vi "VI Tree.vi"   [LabVIEW 2018]
uses:
  app/solar_app_ctl Info.ctl
  excel/solar_excel_ctl TSV.ctl
  excel/solar_excel_ctl App.ctl
  excel/solar_excel_ctl Format.ctl
  excel/solar_excel_ctl Workbook.ctl
  excel/solar_excel_ctl Worksheet.ctl
  misc/solar_misc_ctl Email Config.ctl
  qtimer/solar_qtimer_ctl QTimer Settings.ctl
  qtimer/solar_qtimer_ctl QTimer.ctl
  qtimer/solar_qtimer_ctl Refnum.ctl
  qtimer/solar_qtimer_ctl SEQ.ctl
  solar/solar.lvclass
  voyager/solar_voy_ctl Voyager Refnum.ctl
  solar/solar_ctl Target Global.ctl
  solar/solar_ctl SOLAR Global.ctl
  solar/solar_ctl SOLAR Refnum.ctl
  solar/solar_ctl SOLAR UI Panes.ctl
  tcp/solar_tcp_ctl Action.ctl
  tcp/solar_tcp_ctl Config.ctl
  tcp/solar_tcp_ctl Debug.ctl
  tcp/solar_tcp_ctl Data.ctl
  type/solar_type Item Type.ctl
  type/solar_type Item.ctl
  voyager/solar_voy_def/solar_voy_def_ctl HANDSHAKE.ctl
  voyager/solar_voy_def/solar_voy_def_ctl ITEM TYPE.ctl
  voyager/solar_voy_def/solar_voy_def_ctl ITEM.ctl
  voyager/solar_voy_def/solar_voy_def_ctl HDR.ctl
  voyager/solar_voy_def/solar_voy_def_ctl INTERFACE (LINC).ctl
  voyager/solar_voy_def/solar_voy_def_ctl INTERFACE.ctl
  voyager/solar_voy_def/solar_voy_def_ctl ITEM (Simple).ctl
  voyager/solar_voy_def/solar_voy_def_ctl MODIFIERS CONVERSION.ctl
  voyager/solar_voy_def/solar_voy_def_ctl MODIFIERS LIMITS.ctl
  voyager/solar_voy_def/solar_voy_def_ctl MODIFIERS STATE.ctl
  voyager/solar_voy_def/solar_voy_def_ctl MODIFIERS UNITS.ctl
  voyager/solar_voy_def/solar_voy_def_ctl MODIFIERS.ctl
  voyager/solar_voy_def/solar_voy_def_ctl PACKET_ID.ctl
  voyager/solar_voy_def/solar_voy_def_ctl PACKET.ctl
  voyager/solar_voy_def/solar_voy_def_ctl PATH.ctl
  voyager/solar_voy_ctl Port Setup.ctl
  voyager/solar_voy_ctl Port.ctl
  voyager/solar_voy_ctl Setup.ctl
  voyager/solar_voy_ctl TCP.ctl
  voyager/solar_voy_ctl Voyager.ctl
types:
  T1 = cluster{"Native COSMOS Packets":cluster{"MYUINT8":cluster{"VALUE":u8}, "MYUINT16":cluster{"VALUE":u16}, "MYUINT32":cluster{"VALUE":u32}, "MYUINT64":cluster{"VALUE":u64}, "MYINT8":cluster{"VALUE":i8}, "MYINT16":cluster{"VALUE":i16}, "MYINT32":cluster{"VALUE":i32}, "MYINT64":cluster{"VALUE":i64}, "MYFLOAT32":cluster{"VALUE":sgl}, "MYFLOAT64":cluster{"VALUE":dbl}, "MYSTRING":cluster{"VALUE":string}, "MYBLOCK":cluster{"VALUE,t=block":string}}, "Native COSMOS Array Packets":cluster{"MYUINT8_1D":cluster{"VALUE":u8[]}, "MYUINT16_1D":cluster{"VALUE":u16[]}, "MYUINT32_1D":cluster{"VALUE":u32[]}, "MYUINT64_1D":cluster{"VALUE":u64[]}, "MYINT8_1D":cluster{"VALUE":i8[]}, "MYINT16_1D":cluster{"VALUE":i16[]}, "MYINT32_1D":cluster{"VALUE":i32[]}, "MYINT64_1D":cluster{"VALUE":i64[]}, "MYFLOAT32_1D":cluster{"VALUE":sgl[]}, "MYFLOAT64_1D":cluster{"VALUE":dbl[]}, "MYSTRING_1D":cluster{"VALUE":string[]}, "MYBLOCK_1D":cluster{"VALUE,t=block":string[]}}, "Native COSMOS Array Packets Fixed":cluster{"MYUINT8_1D":cluster{"VALUE,b=24":u8[]}, "MYUINT16_1D":cluster{"VALUE,b=48":u16[]}, "MYUINT32_1D":cluster{"VALUE,b=96":u32[]}, "MYUINT64_1D":cluster{"VALUE,b=192":u64[]}, "MYINT8_1D":cluster{"VALUE,b=24":i8[]}, "MYINT16_1D":cluster{"VALUE,b=48":i16[]}, "MYINT32_1D":cluster{"VALUE,b=96":i32[]}, "MYINT64_1D":cluster{"VALUE,b=192":i64[]}, "MYFLOAT32_1D":cluster{"VALUE,b=128":sgl[]}, "MYFLOAT64_1D":cluster{"VALUE,b=256":dbl[]}, "MYSTRING_1D":cluster{"VALUE,b=352,e=88":string[]}, "MYBLOCK_1D":cluster{"VALUE,t=block,b=192,e=48":string[]}}, "Custom LabVIEW Packets":cluster{"MYUINT8_ENUM":cluster{"VALUE":enum8{"ITEM1", "ITEM2", "ITEM3"}}, "MYUINT16_ENUM":cluster{"VALUE":enum16{"CAT", "DOG", "BIRD", "MOOSE"}}, "MYUINT32_ENUM":cluster{"VALUE":enum32{"ryan", "susan", "steve", "larry", "smith", "joe"}}, "MYBOOLEAN":cluster{"VALUE,s=OFF|ON":bool}, "MYSTRING_FIXED":cluster{"VALUE,b=24":string}, "MYBLOCK_FIXED":cluster{"VALUE,t=block,b=32":string}, "MYPATH":cluster{"VALUE":path}}, "Custom Test Packets":cluster{"MYTEST1":cluster{"MYFLOAT64":dbl, "MYSTRING":string}, "MYTEST2":cluster{"MYFLOAT64":dbl, "MYBLOCK,t=block":string}, "MYTEST3":cluster{"MYBOOLEAN,s=OK|ERROR":bool, "MYI32":i32, "MYSTRING":string}, "TEST_PACKET":cluster{"U32_COUNTER":u32, "DBL_NUMBER":dbl, "STRING,b=480":string, "BOOLEAN":bool, "U16_ENUM":enum16{"ENUM_ONE", "ENUM_TWO", "ENUM_THREE"}, "U8_RING":u8, "U32_ARRAY,e=5":u32[], "U8":u32}}}
  T2 = typedef "solar_voy_ctl Voyager.ctl" = cluster{"PACKETS":T3[], "COSMOS_Root":path, "CMD_HDR":T8, "TLM_HDR":T8, "TCPs":T9[], "VoyagerIDOffset":cluster{"VoyagerIDOffset":u16[], "Target Names":string[]}}
  T3 = typedef "solar_voy_def_ctl PACKET.ctl" = cluster{"PACKET_ID":T4, "ENDIAN":enum8{"BIG", "LITTLE"}, "DESC":string, "HZRD":bool, "ITEMS":T5[], "NoExport":bool, "last_time":timestamp, "last_count":u32, "last_data":string}
  T4 = typedef "solar_voy_def_ctl PACKET_ID.ctl" = cluster{"ID":u16, "CMD":enum8{"CMD", "TLM"}, "TARGET":string, "PACKET":string}
  T5 = typedef "solar_voy_def_ctl ITEM.ctl" = cluster{"NAME":string, "OFFSET":i32, "SIZE":i32, "TYPE":T6, "EACH_SIZE":i32, "LVTYPE":T7, "MIN":dbl, "MAX":dbl, "DEFAULT":string, "DESC":string, "ID":bool, "MODIFIERS":variant, "last_value":variant}
  T6 = typedef "solar_voy_def_ctl ITEM TYPE.ctl" = enum8{"BLOCK", "INT", "UINT", "FLOAT", "STRING"}
  T7 = typedef "solar_type Item Type.ctl" = enum16{"NULL", "UNKNOWN", "CLUSTER", "I8", "I16", "I32", "I64", "U8", "U16", "U32", "U64", "U8_ENUM", "U16_ENUM", "U32_ENUM", "SGL", "DBL", "BOOLEAN", "STRING", "PATH", "VISA", "TAG", "TIME", "I8_1D", "I16_1D", "I32_1D", "I64_1D", "U8_1D", "U16_1D", "U32_1D", "U64_1D", "U8_ENUM_1D", "U16_ENUM_1D", "U32_ENUM_1D", "SGL_1D", "DBL_1D", "BOOLEAN_1D", "STRING_1D", "PATH_1D", "VISA_1D", "TAG_1D", "TIME_1D", "I8_2D", "I16_2D", "I32_2D", "I64_2D", "U8_2D", "U16_2D", "U32_2D", "U64_2D", "U8_ENUM_2D", "U16_ENUM_2D", "U32_ENUM_2D", "SGL_2D", "DBL_2D", "BOOLEAN_2D", "STRING_2D", "PATH_2D", "VISA_2D", "TAG_2D", "TIME_2D"}
  T8 = typedef "solar_voy_def_ctl HDR.ctl" = cluster{"ITEMS":T5[], "LENGTH_NAME":string, "LENGTH_VALUE_OFFSET":i32, "ID_NAME":string, "ENDIAN":enum8{"BIG", "LITTLE"}, "GUID_NAME":string, "DEFAULT_TARGET":string, "DEFAULT_PACKET":string, "DEFAULT_ERROR":string}
  T9 = typedef "solar_voy_ctl TCP.ctl" = cluster{"Connected":bool, "Port":u16, "Listener":refnum<k5>, "ServerIP":string, "TCP":refnum<k5>, "Setup":T10, "VIRefnum":refnum<vi>, "TARGETS_CMD":string[], "TARGETS_TLM":string[]}
  T10 = typedef "solar_voy_ctl Port Setup.ctl" = enum8{"SERVER", "CLIENT", "SERVER_CMD", "SERVER_TLM"}
  T11 = typedef "solar_voy_ctl Voyager Refnum.ctl" = refnum<k1>
  T12 = typedef "solar_voy_ctl Setup.ctl" = cluster{"HEADER":enum8{"LINC", "CCSDS"}, "COSMOS_ROOT":path, "DEFAULT_TARGET":string}
  T13 = typedef "solar_voy_ctl Port.ctl" = cluster{"Setup":T10, "Port":u16, "ServerIP":string, "Target":string}
  T14 = typedef "solar_voy_def_ctl PATH.ctl" = enum8{"..", "config", "config/data", "config/system", "config/targets", "config/targets/TARGET", "config/targets/TARGET/cmd_tlm", "config/targets/TARGET/lib", "config/targets/TARGET/screens", "config/tools", "config/tools/cmd_tlm_server", "config/tools/data_viewer", "config/tools/handbook_creator", "config/tools/launcher", "config/tools/limits_monitor", "config/tools/opengl_builder", "config/tools/script_runner", "config/tools/table_manager", "config/tools/test_runner", "config/tools/tlm_extractor", "config/tools/tlm_grapher", "config/tools/tlm_viewer", "lib", "outputs", "outputs/handbooks", "outputs/logs", "outputs/saved_config", "outputs/tables", "outputs/tmp", "procedures", "tools", "Launcher.bat", "config/system/system.txt", "config/targets/TARGET/cmd_tlm/TARGET_cmd.txt", "config/targets/TARGET/cmd_tlm/TARGET_tlm.txt", "config/targets/TARGET/cmd_tlm_server.txt", "config/targets/TARGET/target.txt", "config/tools/cmd_tlm_server/cmd_tlm_server.txt", "config/tools/data_viewer/data_viewer.txt", "config/tools/handbook_creator/handbook_creator.txt", "config/tools/launcher/launcher.txt", "config/tools/limits_monitor/limits_monitor.txt", "config/tools/opengl_builder/opengl_builder.txt", "config/tools/script_runner/script_runner.txt", "config/tools/table_manager/table_manager.txt", "config/tools/test_runner/test_runner.txt", "config/tools/tlm_extractor/tlm_extractor.txt", "config/tools/tlm_grapher/tlm_grapher.txt", "config/tools/tlm_viewer/tlm_viewer.txt"}
  T15 = typedef "solar_voy_def_ctl MODIFIERS.ctl" = cluster{"LIMITS":T16, "UNITS":T17, "STATES":T18[], "CONVERSION":T19, "FORMAT":string, "REQUIRED":bool, "META":string[][]}
  T16 = typedef "solar_voy_def_ctl MODIFIERS LIMITS.ctl" = cluster{"NAME":string, "PERSIST":i32, "EN":bool, "RED_LO":dbl, "YEL_LO":dbl, "YEL_HI":dbl, "RED_HI":dbl, "GRN_LO":dbl, "GRN_HI":dbl, "FILENAME":string, "ARGS":string}
  T17 = typedef "solar_voy_def_ctl MODIFIERS UNITS.ctl" = cluster{"FULL":string, "ABV":string}
  T18 = typedef "solar_voy_def_ctl MODIFIERS STATE.ctl" = cluster{"KEY":string, "VALUE":string, "COLOR":string, "DESC":string, "HZRD":bool}
  T19 = typedef "solar_voy_def_ctl MODIFIERS CONVERSION.ctl" = cluster{"GENERIC":string, "FILENAME":string, "ARGS":string, "POLYS":cluster{"SEG":bool, "POLY":dbl[]}[]}
  T20 = typedef "solar_voy_def_ctl ITEM (Simple).ctl" = cluster{"NAME":string, "LVTYPE":T7, "BIT_SIZE":i32, "TYPE":T6, "DEFAULT":string, "EACH_SIZE":i32, "ID":bool, "STATES(k,v)":string[][], "DESC":string}
  T21 = typedef "solar_voy_def_ctl INTERFACE.ctl" = cluster{"INTERFACE":string, "TARGETS":string[], "Other":string[]}
  T22 = typedef "solar_voy_def_ctl INTERFACE (LINC).ctl" = cluster{"name":string, "hostname":string, "port":u16, "handshake_enabled":bool, "response_timeout":dbl, "read_timeout":dbl, "write_timeout":dbl, "length_bitoffset":i32, "length_bitsize":i32, "length_value_offset":i32, "fieldname_guid":string, "endianness":enum8{"BIG", "LITTLE"}, "fieldname_cmd_length":string, "Targets":string[]}
  T23 = typedef "solar_voy_def_ctl HANDSHAKE.ctl" = cluster{"ORIGIN":enum8{"RMT", "LCL"}, "STATUS,s=OK,ERROR":bool, "CODE":i32, "TIME_SECONDS":u32, "TIME_MICROSECONDS":u32, "DATA,t=BLOCK":string}
  T24 = typedef "solar_type Item.ctl" = cluster{"Item":string, "Type":T7, "Value":variant, "States":string[]}
  T25 = cluster{"U8":u8, "U16":u16, "U32":u32, "U64":u64, "I8":i8, "I16":i16, "I32":i32, "I64":i64, "U8_ENUM":enum8{"ITEM1", "ITEM2", "ITEM3"}, "U16_ENUM":enum16{"ITEM1", "ITEM2", "ITEM3"}, "U32_ENUM":enum32{"ITEM1", "ITEM2", "ITEM3"}, "SGL":sgl, "DBL":dbl, "BOOLEAN":bool, "STRING":string, "PATH":path, "VISA":refnum<visa-resource-name>, "TAG":tag, "TIME":timestamp, "U8_1D":u8[], "U16_1D":u16[], "U32_1D":u32[], "U64_1D":u64[], "I8_1D":i8[], "I16_1D":i16[], "I32_1D":i32[], "I64_1D":i64[], "U8_ENUM_1D":enum8{"ITEM1", "ITEM2", "ITEM3"}[], "U16_ENUM_1D":enum16{"ITEM1", "ITEM2", "ITEM3"}[], "U32_ENUM_1D":enum32{"ITEM1", "ITEM2", "ITEM3"}[], "SGL_1D":sgl[], "DBL_1D":dbl[], "STRING_1D":string[], "PATH_1D":path[], "VISA_1D":refnum<visa-resource-name>[], "TAG_1D":tag[], "TIME_1D":timestamp[], "U8_2D":u8[][], "U16_2D":u16[][], "U32_2D":u32[][], "U64_2D":u64[][], "I8_2D":i8[][], "I16_2D":i16[][], "I32_2D":i32[][], "I64_2D":i64[][], "U8_ENUM_2D":enum8{"ITEM1", "ITEM2", "ITEM3"}[][], "U16_ENUM_2D":enum16{"ITEM1", "ITEM2", "ITEM3"}[][], "U32_ENUM_2D":enum32{"ITEM1", "ITEM2", "ITEM3"}[][], "SGL_2D":sgl[][], "DBL_2D":dbl[][], "STRING_2D":string[][], "PATH_2D":path[][], "VISA_2D":refnum<visa-resource-name>[][], "TAG_2D":tag[][], "TIME_2D":timestamp[][]}
  T26 = typedef "solar_tcp_ctl Debug.ctl" = cluster{"Time":timestamp, "Action":T27, "ID":string, "Message":string, "Error":string, "Clients":string}
  T27 = typedef "solar_tcp_ctl Action.ctl" = enum16{"Decide", "CreateListener", "Open", "Read", "Write", "Close", "Shutdown", "Done", "ChangePort"}
  T28 = typedef "solar_tcp_ctl Data.ctl" = cluster{"Connected":bool, "Config":T29, "Clients":cluster{"Address":string, "Port":u16, "Valid":bool, "ClientID":refnum<k5>}[], "ConnectionID":refnum<k5>, "Debug":T26[]}
  T29 = typedef "solar_tcp_ctl Config.ctl" = cluster{"TCPServer":enum8{"SERVER", "CLIENT"}, "ServerPort":u16, "IPAddress":string, "ClientPort":u16, "HdrSizeBytes":i32, "HdrLenSubtractBytes":i32, "HdrLenOffsetBits":i32, "HdrLenSizeBits":i32}
  T30 = typedef "solar_ctl Target Global.ctl" = cluster{"Target":string, "Q":refnum<queue>, "UE":refnum<user-event>, "VI":refnum<vi>, "Menu":refnum<k9>, "Data":refnum<data-value>, "Attributes":variant}
  T31 = typedef "solar_ctl SOLAR UI Panes.ctl" = cluster{"Status":bool, "Emergency":bool, "Targets":bool}
  T32 = typedef "solar_ctl SOLAR Refnum.ctl" = refnum<k1>
  T33 = typedef "solar_ctl SOLAR Global.ctl" = cluster{"Targets":T30[], "AppDir":path, "solar.ini":path, "ConfigsDir":path, "CosmosDir":path, "LogsDir":path, "ExePath":path, "ExeVersion":string, "PartNum":string, "AppSetup":string, "Title":string, "Main.ini":path, "Temp.ini":path, "vSOLAR":string, "Splash.png":string, "SplashWait":i32, "SOLARUE":refnum<user-event>, "VoyagerRefnum":T11, "QTimerRefnum":T34}
  T34 = typedef "solar_qtimer_ctl Refnum.ctl" = refnum<k1>
  T35 = typedef "solar_qtimer_ctl SEQ.ctl" = cluster{"QTimers":T36[]}
  T36 = typedef "solar_qtimer_ctl QTimer.ctl" = cluster{"Settings":T37, "Queue":refnum<queue>, "QTimerQ":refnum<queue>, "VI Refnum":refnum<vi>}
  T37 = typedef "solar_qtimer_ctl QTimer Settings.ctl" = cluster{"QTimer":string, "Delay":i32, "Start":bool, "EnQ_Type":enum8{"Normal", "Priority", "IgnoreIfExists"}, "Messages":cluster{"MSG":string, "DATA":variant}[]}
  T38 = typedef "solar_misc_ctl Email Config.ctl" = cluster{"Enabled":bool, "MailServer":string, "MailServerPort":u16, "EmailTimeout":i32, "ReturnAddress":string, "Recipients":string[], "Subject":string}
  T39 = typedef "solar_excel_ctl Worksheet.ctl" = cluster{"ExcelApp":refnum<k7>, "Workbooks":refnum<k7>, "TSV":refnum<queue>, "OpenWkb":refnum<k7>, "Worksheets":refnum<k7>, "OpenWksh":refnum<k7>}
  T40 = typedef "solar_excel_ctl Workbook.ctl" = cluster{"ExcelApp":refnum<k7>, "Workbooks":refnum<k7>, "TSV":refnum<queue>, "OpenWkb":refnum<k7>}
  T41 = typedef "solar_excel_ctl TSV.ctl" = cluster{"Path":path, "Dirty":bool, "ActiveSheet":u8, "Worksheets":string[], "Worksheet Cells":cluster{"Cells":string[][]}[]}
  T42 = typedef "solar_excel_ctl Format.ctl" = cluster{"Set Cell Color":bool, "Cell Color":u32, "Set Text Color":bool, "Text Color":u32, "Set Text Style":bool, "Text Style":enum8{"Plain", "Bold", "Italic"}}
  T43 = typedef "solar_excel_ctl App.ctl" = cluster{"ExcelApp":refnum<k7>, "Workbooks":refnum<k7>, "TSV":refnum<queue>}
  T44 = typedef "solar_app_ctl Info.ctl" = cluster{"AppName":string, "AppDir":path, "solar.ini":path, "ConfigsDir":path, "LogsDir":path, "CosmosDir":path, "ExePath":path, "vApp":string, "Part":string, "Setup":string, "Title":string, "Main.ini":path, "temp.ini":path, "vSOLAR":string, "Splash.png":string}
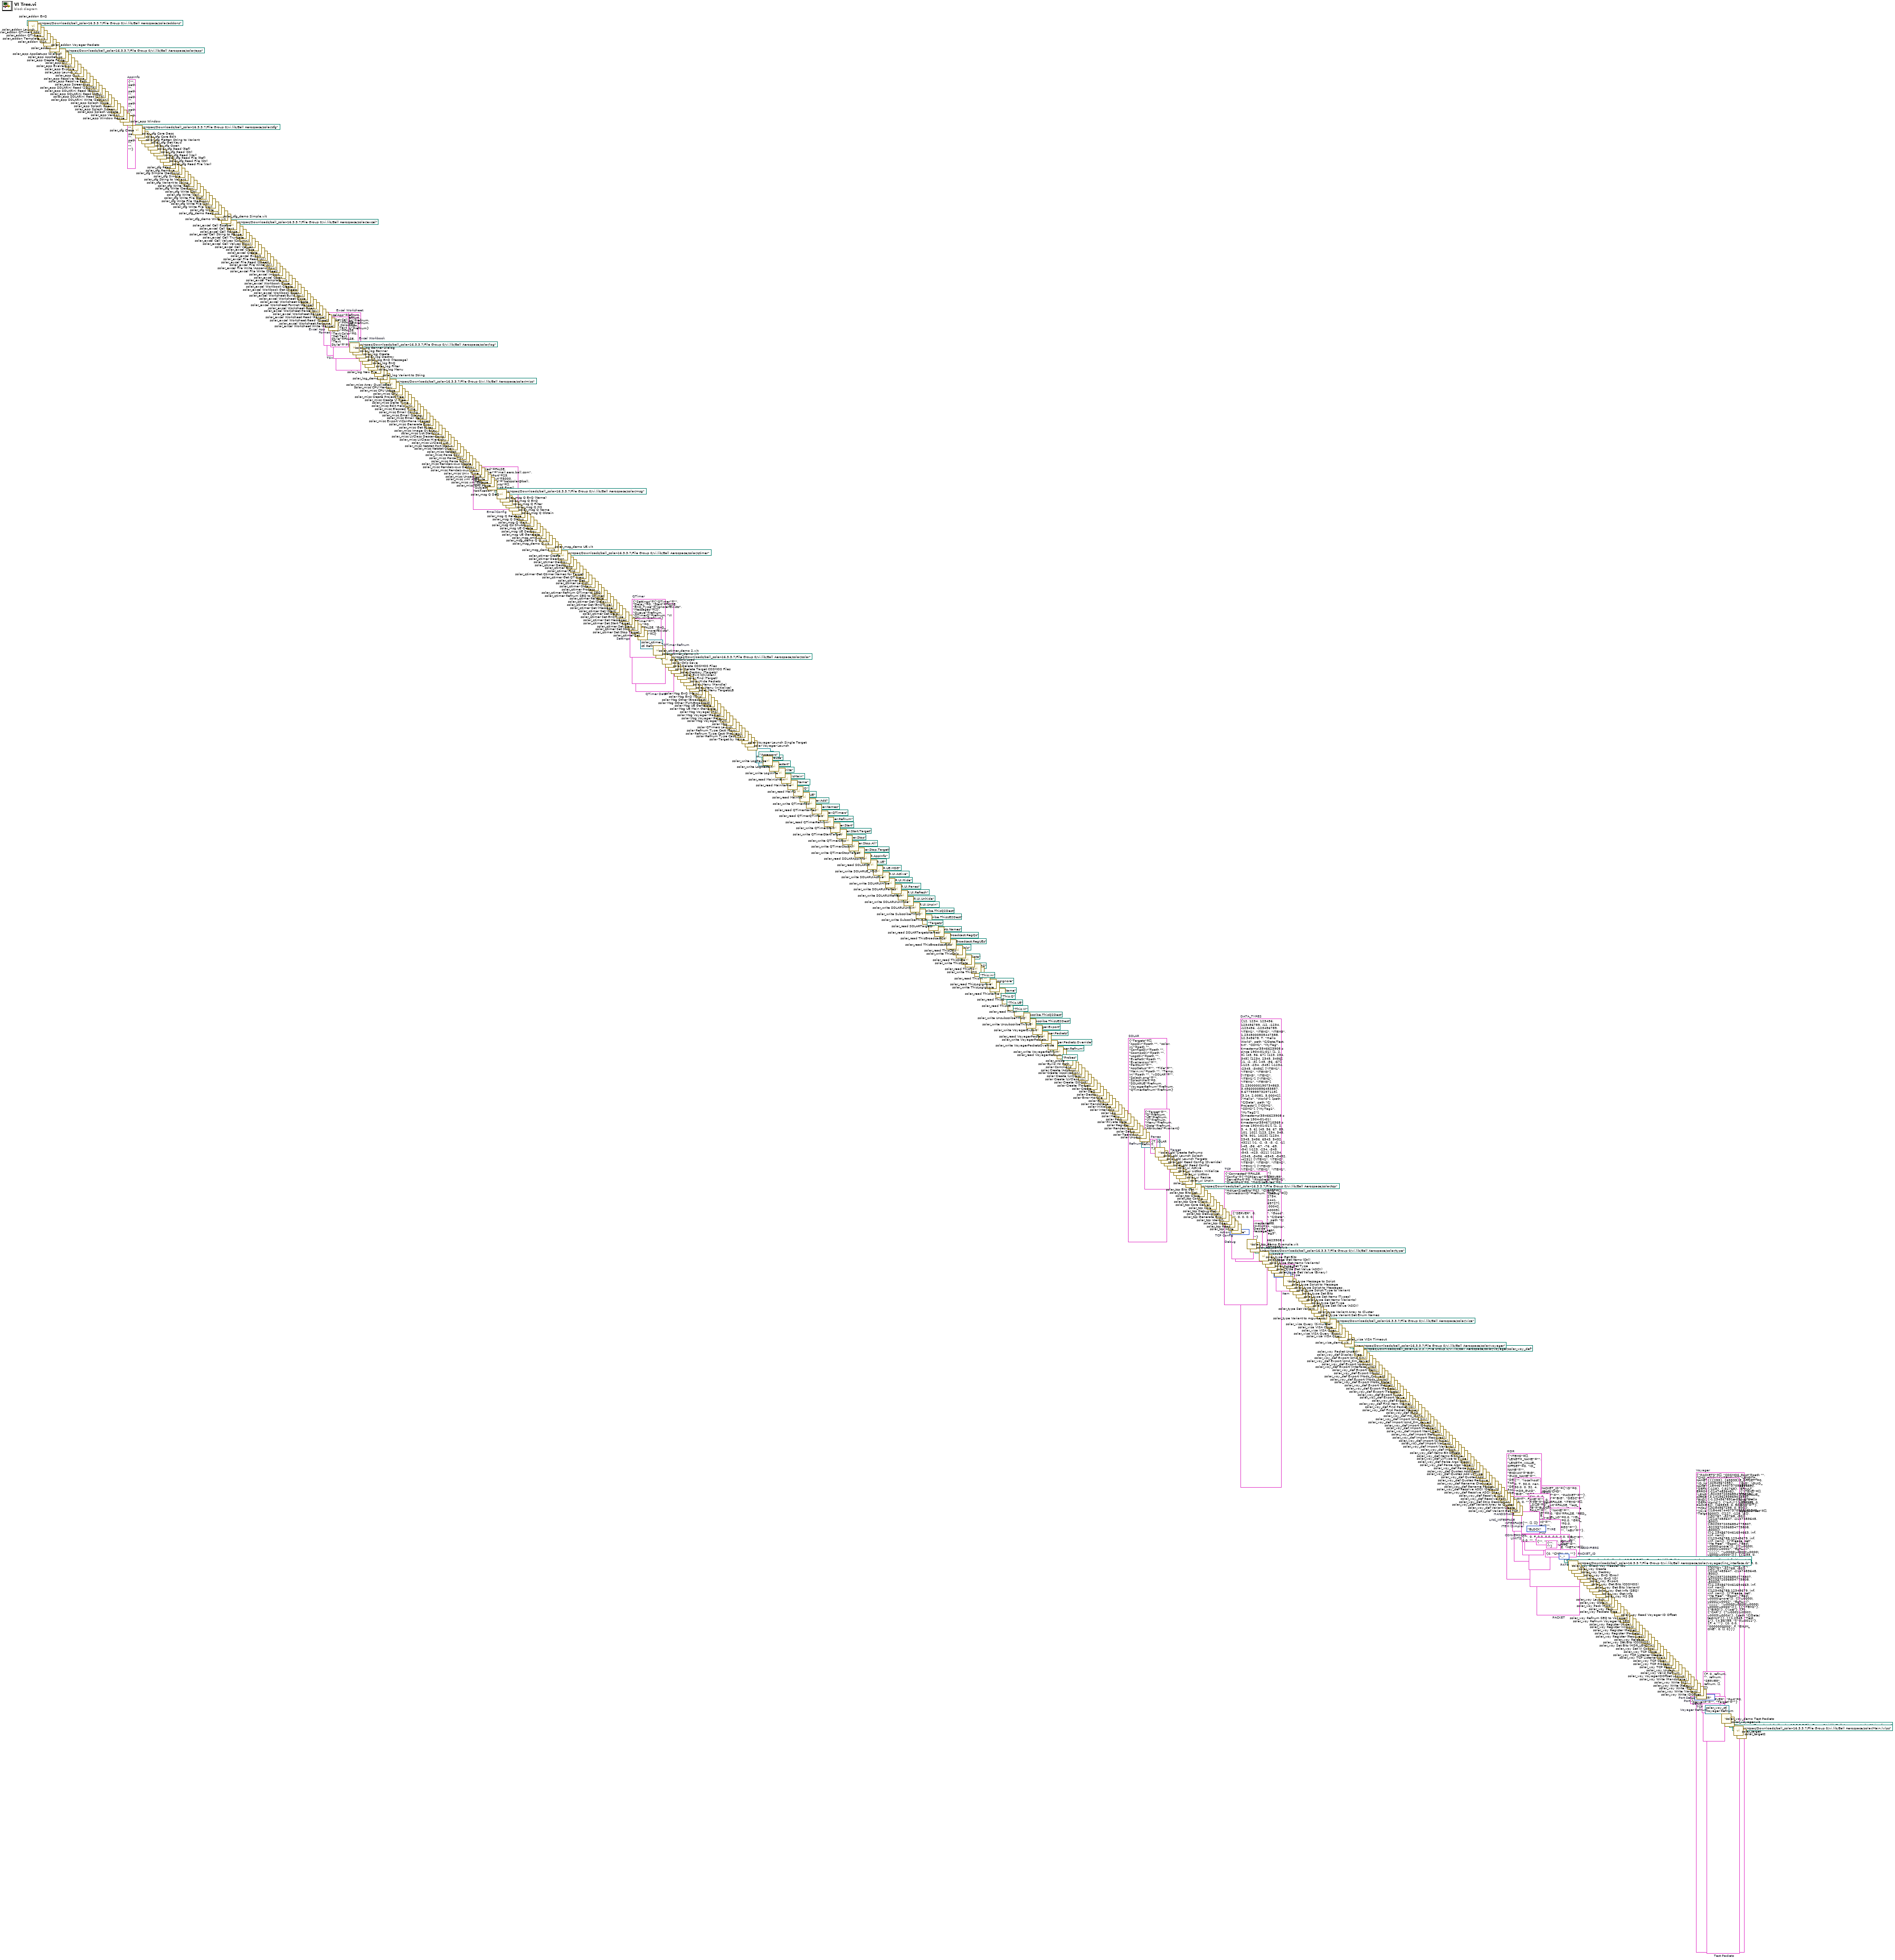
[diagram p0: block diagram]
diagram:
  (unwired) path "C:/Users/rcpac/Downloads/ball_solar-16.3.3.7/File Group 0/vi.lib/Ball Aerospace/solar/Main.lvlps"
  (unwired) path "C:/Users/rcpac/Downloads/ball_solar-16.3.3.7/File Group 0/vi.lib/Ball Aerospace/solar/Main.aliases"
  (unwired) T1 {"Native COSMOS Packets"={"MYUINT8"={"VALUE"=255}, "MYUINT16"={"VALUE"=65535}, "MYUINT32"={"VALUE"=4294967295}, "MYUINT64"={"VALUE"=18446744073709551615}, "MYINT8"={"VALUE"=-128}, "MYINT16"={"VALUE"=-32768}, "MYINT32"={"VALUE"=-2147483648}, "MYINT64"={"VALUE"=-9223372036854775808}, "MYFLOAT32"={"VALUE"=3.141563}, "MYFLOAT64"={"VALUE"=-1.234567891e-05}, "MYSTRING"={"VALUE"="Hello World"}, "MYBLOCK"={"VALUE,t=block"="Þ­¾ï"}}, "Native COSMOS Array Packets"={"MYUINT8_1D"={"VALUE"=[255, 0, 5]}, "MYUINT16_1D"={"VALUE"=[65535, 0, 50]}, "MYUINT32_1D"={"VALUE"=[4294967295, 0, 500]}, "MYUINT64_1D"={"VALUE"=[18446744073709551615, 0, 5000]}, "MYINT8_1D"={"VALUE"=[127, -128, -5]}, "MYINT16_1D"={"VALUE"=[32767, -32768, -50]}, "MYINT32_1D"={"VALUE"=[2147483647, -2147483648, -500]}, "MYINT64_1D"={"VALUE"=[9223372036854775807, -9223372036854775808, -5000]}, "MYFLOAT32_1D"={"VALUE"=[-1.234567, inf, -inf, nan]}, "MYFLOAT64_1D"={"VALUE"=[123456789.12345679, inf, -inf, nan]}, "MYSTRING_1D"={"VALUE"=["Please, set", "Me Free", "Good", "Bad\u0000ignore"]}, "MYBLOCK_1D"={"VALUE,t=block"=["\u0000\u0001\u0002", "Eg‰«Íï", "ÿÿÿÿ", "\u0000\u0000\u0000\u0000\u0000"]}}, "Native COSMOS Array Packets Fixed"={"MYUINT8_1D"={"VALUE,b=24"=[255, 0, 5]}, "MYUINT16_1D"={"VALUE,b=48"=[65535, 0, 50]}, "MYUINT32_1D"={"VALUE,b=96"=[4294967295, 0, 500]}, "MYUINT64_1D"={"VALUE,b=192"=[18446744073709551615, 0, 5000]}, "MYINT8_1D"={"VALUE,b=24"=[127, -128, -5]}, "MYINT16_1D"={"VALUE,b=48"=[32767, -32768, -50]}, "MYINT32_1D"={"VALUE,b=96"=[2147483647, -2147483648, -500]}, "MYINT64_1D"={"VALUE,b=192"=[9223372036854775807, -9223372036854775808, -5000]}, "MYFLOAT32_1D"={"VALUE,b=128"=[-1.234567, inf, -inf, nan]}, "MYFLOAT64_1D"={"VALUE,b=256"=[123456789.12345679, inf, -inf, nan]}, "MYSTRING_1D"={"VALUE,b=352,e=88"=["Please, set", "Me Free", "Good", "Bad\u0000ignore"]}, "MYBLOCK_1D"={"VALUE,t=block,b=192,e=48"=["\u0000\u0001\u0002", "Eg‰«Íï", "ÿÿÿÿ", "\u0000\u0000\u0000\u0000\u0000"]}}, "Custom LabVIEW Packets"={"MYUINT8_ENUM"={"VALUE"=enum."ITEM2"}, "MYUINT16_ENUM"={"VALUE"=enum."BIRD"}, "MYUINT32_ENUM"={"VALUE"=enum."joe"}, "MYBOOLEAN"={"VALUE,s=OFF|ON"=FALSE}, "MYSTRING_FIXED"={"VALUE,b=24"="CAR"}, "MYBLOCK_FIXED"={"VALUE,t=block,b=32"="\u0001\u0002\u0003\u0004"}, "MYPATH"={"VALUE"=path "C:/Data/test.txt"}}, "Custom Test Packets"={"MYTEST1"={"MYFLOAT64"=1.2345, "MYSTRING"="Test 1"}, "MYTEST2"={"MYFLOAT64"=4.56789, "MYBLOCK,t=block"="º^º\u0011"}, "MYTEST3"={"MYBOOLEAN,s=OK|ERROR"=FALSE, "MYI32"=4, "MYSTRING"=""}, "TEST_PACKET"={"U32_COUNTER"=0, "DBL_NUMBER"=0.0, "STRING,b=480"="0000000000", "BOOLEAN"=FALSE, "U16_ENUM"=enum."ENUM_ONE", "U8_RING"=0, "U32_ARRAY,e=5"=[], "U8"=0}}}  # Test Packets
  (unwired) T2 {"PACKETS"=[], "COSMOS_Root"=path "", "CMD_HDR"={"ITEMS"=[], "LENGTH_NAME"="", "LENGTH_VALUE_OFFSET"=0, "ID_NAME"="", "ENDIAN"=enum."BIG", "GUID_NAME"="", "DEFAULT_TARGET"="", "DEFAULT_PACKET"="", "DEFAULT_ERROR"=""}, "TLM_HDR"={"ITEMS"=[], "LENGTH_NAME"="", "LENGTH_VALUE_OFFSET"=0, "ID_NAME"="", "ENDIAN"=enum."BIG", "GUID_NAME"="", "DEFAULT_TARGET"="", "DEFAULT_PACKET"="", "DEFAULT_ERROR"=""}, "TCPs"=[], "VoyagerIDOffset"={"VoyagerIDOffset"=[], "Target Names"=[]}}  # Voyager
  (unwired) T11 refnum items=["voyager"]  # Voyager Refnum
  (unwired) T9 {"Connected"=FALSE, "Port"=0, "Listener"=refnum, "ServerIP"="", "TCP"=refnum, "Setup"=enum."SERVER", "VIRefnum"=refnum, "TARGETS_CMD"=[], "TARGETS_TLM"=[]}  # TCP
  (unwired) T12 {"HEADER"=enum."LINC", "COSMOS_ROOT"=path "", "DEFAULT_TARGET"=""}  # Setup
  (unwired) T13 {"Setup"=enum."SERVER", "Port"=0, "ServerIP"="", "Target"=""}  # Port
  (unwired) solar_voy_ctl_Port_Setup."SERVER"  # Port Setup
  (unwired) path "C:/Users/rcpac/Downloads/ball_solar-16.3.3.7/File Group 0/vi.lib/Ball Aerospace/solar/voyager/linc_interface.rb"
  (unwired) path "C:/Users/rcpac/Downloads/ball_solar-16.3.3.7/File Group 0/vi.lib/Ball Aerospace/solar/voyager/linc_definitions.txt"
  (unwired) solar_voy_def_ctl_PATH.".."  # PATH
  (unwired) T4 {"ID"=0, "CMD"=enum."CMD", "TARGET"="", "PACKET"=""}  # PACKET_ID
  (unwired) T3 {"PACKET_ID"={"ID"=0, "CMD"=enum."CMD", "TARGET"="", "PACKET"=""}, "ENDIAN"=enum."BIG", "DESC"="", "HZRD"=FALSE, "ITEMS"=[], "NoExport"=FALSE, "last_time"=timestamp(0 s since 1904-01-01), "last_count"=0, "last_data"=""}  # PACKET
  (unwired) T15 {"LIMITS"={"NAME"="", "PERSIST"=0, "EN"=FALSE, "RED_LO"=0.0, "YEL_LO"=0.0, "YEL_HI"=0.0, "RED_HI"=0.0, "GRN_LO"=0.0, "GRN_HI"=0.0, "FILENAME"="", "ARGS"=""}, "UNITS"={"FULL"="", "ABV"=""}, "STATES"=[], "CONVERSION"={"GENERIC"="", "FILENAME"="", "ARGS"="", "POLYS"=[]}, "FORMAT"="", "REQUIRED"=FALSE, "META"=[]}  # MODIFIERS
  (unwired) T17 {"FULL"="", "ABV"=""}  # UNITS
  (unwired) T18 {"KEY"="", "VALUE"="", "COLOR"="", "DESC"="", "HZRD"=FALSE}  # STATE
  (unwired) T16 {"NAME"="", "PERSIST"=0, "EN"=FALSE, "RED_LO"=0.0, "YEL_LO"=0.0, "YEL_HI"=0.0, "RED_HI"=0.0, "GRN_LO"=0.0, "GRN_HI"=0.0, "FILENAME"="", "ARGS"=""}  # LIMITS
  (unwired) T19 {"GENERIC"="", "FILENAME"="", "ARGS"="", "POLYS"=[]}  # CONVERSION
  (unwired) T5 {"NAME"="", "OFFSET"=0, "SIZE"=0, "TYPE"=enum."BLOCK", "EACH_SIZE"=0, "LVTYPE"=enum."NULL", "MIN"=0.0, "MAX"=0.0, "DEFAULT"="", "DESC"="", "ID"=FALSE, "MODIFIERS"=variant, "last_value"=variant}  # ITEM
  (unwired) solar_voy_def_ctl_ITEM_TYPE."BLOCK"  # TYPE
  (unwired) T20 {"NAME"="", "LVTYPE"=enum."NULL", "BIT_SIZE"=0, "TYPE"=enum."BLOCK", "DEFAULT"="", "EACH_SIZE"=0, "ID"=FALSE, "STATES(k,v)"=[], "DESC"=""}  # ITEM (Simple)
  (unwired) T21 {"INTERFACE"="", "TARGETS"=[], "Other"=[]}  # INTERFACE
  (unwired) T22 {"name"="", "hostname"="localhost", "port"=0, "handshake_enabled"=TRUE, "response_timeout"=30.0, "read_timeout"=nan, "write_timeout"=30.0, "length_bitoffset"=0, "length_bitsize"=32, "length_value_offset"=4, "fieldname_guid"="HDR_GUID", "endianness"=enum."BIG", "fieldname_cmd_length"="HDR_LENGTH", "Targets"=[]}  # LINC_INTERFACE
  (unwired) T8 {"ITEMS"=[], "LENGTH_NAME"="", "LENGTH_VALUE_OFFSET"=0, "ID_NAME"="", "ENDIAN"=enum."BIG", "GUID_NAME"="", "DEFAULT_TARGET"="", "DEFAULT_PACKET"="", "DEFAULT_ERROR"=""}  # HDR
  (unwired) T23 {"ORIGIN"=enum."RMT", "STATUS,s=OK,ERROR"=FALSE, "CODE"=0, "TIME_SECONDS"=0, "TIME_MICROSECONDS"=0, "DATA,t=BLOCK"=""}  # HANDSHAKE
  (unwired) path "C:/Users/rcpac/Downloads/ball_solar-16.3.3.7/File Group 0/vi.lib/Ball Aerospace/solar/voyager/solar_voy_def"
  (unwired) path "C:/Users/rcpac/Downloads/ball_solar-16.3.3.7/File Group 0/vi.lib/Ball Aerospace/solar/voyager"
  (unwired) path "C:/Users/rcpac/Downloads/ball_solar-16.3.3.7/File Group 0/vi.lib/Ball Aerospace/solar/visa"
  (unwired) T24 {"Item"="", "Type"=enum."NULL", "Value"=variant, "States"=[]}  # Item
  (unwired) solar_type_Item_Type."NULL"  # Type
  (unwired) T25 {"U8"=12, "U16"=1234, "U32"=123456, "U64"=123456789, "I8"=-12, "I16"=-1234, "I32"=-123456, "I64"=-123456789, "U8_ENUM"=enum."ITEM1", "U16_ENUM"=enum."ITEM2", "U32_ENUM"=enum."ITEM3", "SGL"=1.2345, "DBL"=12.345678, "BOOLEAN"=TRUE, "STRING"="Hello World", "PATH"=path "C:/Data/Test.txt", "VISA"="COM1", "TAG"="MyTag", "TIME"=timestamp(3546623908.244 s since 1904-01-01), "U8_1D"=[1, 2, 3], "U16_1D"=[45, 56, 67], "U32_1D"=[123, 234, 345], "U64_1D"=[1234, 2345, 3456], "I8_1D"=[-1, -2, -3], "I16_1D"=[-45, -56, -67], "I32_1D"=[-123, -234, -345], "I64_1D"=[-1234, -2345, -3456], "U8_ENUM_1D"=[enum."ITEM1", enum."ITEM2", enum."ITEM3"], "U16_ENUM_1D"=[enum."ITEM3", enum."ITEM2", enum."ITEM1"], "U32_ENUM_1D"=[enum."ITEM2", enum."ITEM1", enum."ITEM3"], "SGL_1D"=[1.23, 3.456, 5.678], "DBL_1D"=[3.14, 2.0081, 5.00042], "STRING_1D"=["Hello", "World"], "PATH_1D"=[path "C:/Data", path "C:/Projects"], "VISA_1D"=["COM1", "COM2"], "TAG_1D"=["MyTag1", "MyTag2"], "TIME_1D"=[timestamp(3546623908.244 s since 1904-01-01), timestamp(3546710368.244 s since 1904-01-01)], "U8_2D"=[[1, 2, 3], [4, 5, 6]], "U16_2D"=[[45, 56, 67], [89, 101, 102]], "U32_2D"=[[123, 234, 345], [678, 901, 1023]], "U64_2D"=[[1234, 2345, 3456], [6543, 5432, 4321]], "I8_2D"=[[-1, -2, -3], [-3, -2, -1]], "I16_2D"=[[-45, -56, -67], [-76, -65, -54]], "I32_2D"=[[-123, -234, -345], [-543, -423, -321]], "I64_2D"=[[-1234, -2345, -3456], [-6543, -5432, -4231]], "U8_ENUM_2D"=[[enum."ITEM1", enum."ITEM2", enum."ITEM3"], [enum."ITEM3", enum."ITEM2", enum."ITEM1"]], "U16_ENUM_2D"=[[enum."ITEM3", enum."ITEM2", enum."ITEM1"], [enum."ITEM1", enum."ITEM2", enum."ITEM3"]], "U32_ENUM_2D"=[[enum."ITEM2", enum."ITEM1", enum."ITEM3"], [enum."ITEM3", enum."ITEM1", enum."ITEM2"]], "SGL_2D"=[[1.23, 3.456, 5.678], [8.765, 6.543, 3.21]], "DBL_2D"=[[3.14, 2.0081, 5.00042], [4.13, 1.8002, 2.40005]], "STRING_2D"=[["Hello", "World"], ["Good", "Morning"]], "PATH_2D"=[[path "C:/Data", path "C:/Projects"], [path "C:/Test", path "C:/Ball"]], "VISA_2D"=[["COM1", "COM2"], ["COM4", "COM5"]], "TAG_2D"=[["MyTag1", "MyTag2"], ["MyTag3", "MyTag4"]], "TIME_2D"=[[timestamp(3546623908.244 s since 1904-01-01), timestamp(3549392308.244 s since 1904-01-01)], [timestamp(3552074308.244 s since 1904-01-01), timestamp(3554842708.244 s since 1904-01-01)]]}  # DATA_TYPES
  (unwired) path "C:/Users/rcpac/Downloads/ball_solar-16.3.3.7/File Group 0/vi.lib/Ball Aerospace/solar/type"
  (unwired) T26 {"Time"=timestamp(0 s since 1904-01-01), "Action"=enum."Decide", "ID"="", "Message"="", "Error"="", "Clients"=""}  # Debug
  (unwired) T28 {"Connected"=FALSE, "Config"={"TCPServer"=enum."SERVER", "ServerPort"=0, "IPAddress"="", "ClientPort"=0, "HdrSizeBytes"=0, "HdrLenSubtractBytes"=0, "HdrLenOffsetBits"=0, "HdrLenSizeBits"=0}, "Clients"=[], "ConnectionID"=refnum, "Debug"=[]}  # TCP
  (unwired) T29 {"TCPServer"=enum."SERVER", "ServerPort"=0, "IPAddress"="", "ClientPort"=0, "HdrSizeBytes"=0, "HdrLenSubtractBytes"=0, "HdrLenOffsetBits"=0, "HdrLenSizeBits"=0}  # TCP Config
  (unwired) solar_tcp_ctl_Action."Decide"  # Action
  (unwired) path "C:/Users/rcpac/Downloads/ball_solar-16.3.3.7/File Group 0/vi.lib/Ball Aerospace/solar/tcp"
  (unwired) T30 {"Target"="", "Q"=refnum, "UE"=refnum, "VI"=refnum, "Menu"=refnum, "Data"=refnum, "Attributes"=variant}  # Target
  (unwired) T31 {"Status"=TRUE, "Emergency"=TRUE, "Targets"=TRUE}  # Panes
  (unwired) T32 refnum items=["solar"]  # Refnum
  (unwired) T33 {"Targets"=[], "AppDir"=path "", "solar.ini"=path "", "ConfigsDir"=path "", "CosmosDir"=path "", "LogsDir"=path "", "ExePath"=path "", "ExeVersion"="", "PartNum"="", "AppSetup"="", "Title"="", "Main.ini"=path "", "Temp.ini"=path "", "vSOLAR"="", "Splash.png"="", "SplashWait"=0, "SOLARUE"=refnum, "VoyagerRefnum"=refnum, "QTimerRefnum"=refnum}  # SOLAR
  (unwired) path "Probes"
  (unwired) path "Voyager.Refnum"
  (unwired) path "Voyager.Packets.Override"
  (unwired) path "Voyager.Packets"
  (unwired) path "Voyager.Export"
  (unwired) path "Unsubscribe.ThisUE2Dest"
  (unwired) path "Unsubscribe.ThisQ2Dest"
  (unwired) path "This.VI"
  (unwired) path "This.UE"
  (unwired) path "This.Q"
  (unwired) path "This.Name"
  (unwired) path "This.LogIgnore"
  (unwired) path "This.ini"
  (unwired) path "This.HS"
  (unwired) path "This.Data"
  (unwired) path "This.Ctrls"
  (unwired) path "This.Broadcast.RegUEs"
  (unwired) path "This.Broadcast.RegQs"
  (unwired) path "Targets.Names"
  (unwired) path "Targets"
  (unwired) path "Subscribe.ThisUE2Dest"
  (unwired) path "Subscribe.ThisQ2Dest"
  (unwired) path "SOLAR.UI.Unpin"
  (unwired) path "SOLAR.UI.Unhide"
  (unwired) path "SOLAR.UI.Refresh"
  (unwired) path "SOLAR.UI.Panes"
  (unwired) path "SOLAR.UI.Hide"
  (unwired) path "SOLAR.UI.Active"
  (unwired) path "SOLAR.UE.MSG"
  (unwired) path "SOLAR.UE"
  (unwired) path "SOLAR.AppInfo"
  (unwired) path "QTimer.Stop.Target"
  (unwired) path "QTimer.Stop.All"
  (unwired) path "QTimer.Stop"
  (unwired) path "QTimer.Start.Target"
  (unwired) path "QTimer.Start"
  (unwired) path "QTimer.Refnum"
  (unwired) path "QTimer.QTimers"
  (unwired) path "QTimer.Names"
  (unwired) path "QTimer.Add"
  (unwired) path "Main.UE"
  (unwired) path "Main.Q"
  (unwired) path "Main.Name"
  (unwired) path "Main.IsMain"
  (unwired) path "Log.Write"
  (unwired) path "Log.Restart"
  (unwired) path "Log.Pause"
  (unwired) path "Accessors"
  (unwired) refnum<class "solar.lvclass"> refnum ("solar")
  (unwired) refnum<class "solar.lvclass"> refnum ("solar")
  (unwired) path "C:/Users/rcpac/Downloads/ball_solar-16.3.3.7/File Group 0/vi.lib/Ball Aerospace/solar/solar"
  (unwired) T35 {"QTimers"=[]}  # QTimer Data
  (unwired) T34 refnum items=["qtimer"]  # QTimer Refnum
  (unwired) T36 {"Settings"={"QTimer"="", "Delay"=0, "Start"=FALSE, "EnQ_Type"=enum."IgnoreIfExists", "Messages"=[]}, "Queue"=refnum, "QTimerQ"=refnum, "VI Refnum"=refnum}  # QTimer
  (unwired) T37 {"QTimer"="", "Delay"=0, "Start"=FALSE, "EnQ_Type"=enum."IgnoreIfExists", "Messages"=[]}  # Settings
  (unwired) path "C:/Users/rcpac/Downloads/ball_solar-16.3.3.7/File Group 0/vi.lib/Ball Aerospace/solar/qtimer"
  (unwired) path "C:/Users/rcpac/Downloads/ball_solar-16.3.3.7/File Group 0/vi.lib/Ball Aerospace/solar/msg"
  (unwired) T38 {"Enabled"=FALSE, "MailServer"="mail.aero.ball.com", "MailServerPort"=25, "EmailTimeout"=5000, "ReturnAddress"="batcsolar@ball.com", "Recipients"=[], "Subject"="SOLAR Email Notification"}  # EmailConfig
  (unwired) path "C:/Users/rcpac/Downloads/ball_solar-16.3.3.7/File Group 0/vi.lib/Ball Aerospace/solar/misc"
  (unwired) path "C:/Users/rcpac/Downloads/ball_solar-16.3.3.7/File Group 0/vi.lib/Ball Aerospace/solar/log"
  (unwired) T39 {"ExcelApp"=refnum, "Workbooks"=refnum, "TSV"=refnum, "OpenWkb"=refnum, "Worksheets"=refnum, "OpenWksh"=refnum}  # Excel Worksheet
  (unwired) T40 {"ExcelApp"=refnum, "Workbooks"=refnum, "TSV"=refnum, "OpenWkb"=refnum}  # Excel Workbook
  (unwired) T41 {"Path"=path "", "Dirty"=FALSE, "ActiveSheet"=0, "Worksheets"=[], "Worksheet Cells"=[]}  # TSV
  (unwired) T42 {"Set Cell Color"=FALSE, "Cell Color"=0, "Set Text Color"=FALSE, "Text Color"=0, "Set Text Style"=FALSE, "Text Style"=enum."Plain"}  # Format
  (unwired) T43 {"ExcelApp"=refnum, "Workbooks"=refnum, "TSV"=refnum}  # Excel App
  (unwired) path "C:/Users/rcpac/Downloads/ball_solar-16.3.3.7/File Group 0/vi.lib/Ball Aerospace/solar/excel"
  (unwired) path "C:/Users/rcpac/Downloads/ball_solar-16.3.3.7/File Group 0/vi.lib/Ball Aerospace/solar/cfg"
  (unwired) T44 {"AppName"="", "AppDir"=path "", "solar.ini"=path "", "ConfigsDir"=path "", "LogsDir"=path "", "CosmosDir"=path "", "ExePath"=path "", "vApp"="", "Part"="", "Setup"="", "Title"="", "Main.ini"=path "", "temp.ini"=path "", "vSOLAR"="", "Splash.png"=""}  # AppInfo
  (unwired) path "C:/Users/rcpac/Downloads/ball_solar-16.3.3.7/File Group 0/vi.lib/Ball Aerospace/solar/app"
  (unwired) path "C:/Users/rcpac/Downloads/ball_solar-16.3.3.7/File Group 0/vi.lib/Ball Aerospace/solar/addons"
  n1 = call "solar_addon EnQ.vi"() -> ()  [unwired: 11 in, 1 out]
  n2 = call "solar_addon Launch.vi"() -> ()  [unwired: 9 in, 3 out]
  n3 = call "solar_addon QTimers Add.vi"() -> ()  [unwired: 8 in, 4 out]
  n4 = call "solar_addon QTimers.vi"() -> ()  [unwired: 11 in, 1 out]
  n5 = call "solar_addon Template.vit"() -> ()  [unwired: 11 in, 1 out]
  n6 = call "solar_addon VISA.vi"() -> ()  [unwired: 12 in]
  n7 = call "solar_addon Voyager Packets.vi"() -> ()  [unwired: 11 in, 1 out]
  n8 = call "solar_addon.vi"() -> ()  [unwired: 10 in, 2 out]
  n9 = call "solar_app AppSetups (Dialog).vi"() -> ()  [unwired: 11 in, 1 out]
  n10 = call "solar_app AppSetups.vi"() -> ()  [unwired: 11 in, 1 out]
  n11 = call "solar_app Create Folder.vi"() -> ()  [unwired: 10 in, 2 out]
  n12 = call "solar_app Dir.vi"() -> ()  [unwired: 9 in, 3 out]
  n13 = call "solar_app ExeVersion.vi"() -> ()  [unwired: 9 in, 3 out]
  n14 = call "solar_app Explore.vi"() -> ()  [unwired: 11 in, 1 out]
  n15 = call "solar_app Launch VI.vi"() -> ()  [unwired: 10 in, 2 out]
  n16 = call "solar_app Quit.vi"() -> ()  [unwired: 11 in, 1 out]
  n17 = call "solar_app Resolve Name.vi"() -> ()  [unwired: 9 in, 1 out]
  n18 = call "solar_app Resolve Path.vi"() -> ()  [unwired: 8 in, 2 out]
  n19 = call "solar_app Screenshot.vi"() -> ()  [unwired: 9 in, 3 out]
  n20 = call "solar_app SOLARini Read (2DSTR).vi"() -> ()  [unwired: 10 in, 2 out]
  n21 = call "solar_app SOLARini Read (BOOL).vi"() -> ()  [unwired: 10 in, 2 out]
  n22 = call "solar_app SOLARini Read (DBL).vi"() -> ()  [unwired: 10 in, 2 out]
  n23 = call "solar_app SOLARini Read (STR).vi"() -> ()  [unwired: 10 in, 2 out]
  n24 = call "solar_app SOLARini Write (Section).vi"() -> ()  [unwired: 11 in, 1 out]
  n25 = call "solar_app Splash Close.vi"() -> ()  [unwired: 11 in, 1 out]
  n26 = call "solar_app Splash Open.vi"() -> ()  [unwired: 10 in, 2 out]
  n27 = call "solar_app Splash Screen.vi"() -> ()  [unwired: 12 in]
  n28 = call "solar_app Splash Update.vi"() -> ()  [unwired: 10 in, 2 out]
  n29 = call "solar_app Version.vi"() -> ()  [unwired: 11 in, 1 out]
  n30 = call "solar_app Window Resize.vi"() -> ()  [unwired: 9 in, 3 out]
  n31 = call "solar_app Window.vi"() -> ()  [unwired: 11 in, 1 out]
  n32 = call "solar_cfg Close.vi"() -> ()  [unwired: 14 in, 2 out]
  n33 = call "solar_cfg Core Desc.vi"() -> ()  [unwired: 11 in, 1 out]
  n34 = call "solar_cfg Core Edit.vi"() -> ()  [unwired: 7 in, 5 out]
  n35 = call "solar_cfg Flatten String to Variant.vi"() -> ()  [unwired: 9 in, 3 out]
  n36 = call "solar_cfg Get Keys.vi"() -> ()  [unwired: 12 in, 4 out]
  n37 = call "solar_cfg Open.vi"() -> ()  [unwired: 12 in, 4 out]
  n38 = call "solar_cfg Read (Ref).vi"() -> ()  [unwired: 12 in, 4 out]
  n39 = call "solar_cfg Read (Str).vi"() -> ()  [unwired: 12 in, 4 out]
  n40 = call "solar_cfg Read (Var).vi"() -> ()  [unwired: 12 in, 4 out]
  n41 = call "solar_cfg Read File (Ref).vi"() -> ()  [unwired: 13 in, 3 out]
  n42 = call "solar_cfg Read File (Str).vi"() -> ()  [unwired: 12 in, 4 out]
  n43 = call "solar_cfg Read File (Var).vi"() -> ()  [unwired: 12 in, 4 out]
  n44 = call-poly "solar_cfg Read.vi"() -> ()  [unwired: 12 in, 4 out]
  n45 = call "solar_cfg Remove.vi"() -> ()  [unwired: 13 in, 3 out]
  n46 = call "solar_cfg Simple (Sections).vi"() -> ()  [unwired: 8 in, 4 out]
  n47 = call "solar_cfg Simple.vi"() -> ()  [unwired: 8 in, 4 out]
  n48 = call "solar_cfg String to Variant.vi"() -> ()  [unwired: 9 in, 3 out]
  n49 = call "solar_cfg Variant to String.vi"() -> ()  [unwired: 8 in, 4 out]
  n50 = call "solar_cfg Write (Ref).vi"() -> ()  [unwired: 13 in, 3 out]
  n51 = call "solar_cfg Write (Section).vi"() -> ()  [unwired: 13 in, 3 out]
  n52 = call "solar_cfg Write (Str).vi"() -> ()  [unwired: 13 in, 3 out]
  n53 = call "solar_cfg Write (Var).vi"() -> ()  [unwired: 13 in, 3 out]
  n54 = call "solar_cfg Write File (Ref).vi"() -> ()  [unwired: 13 in, 3 out]
  n55 = call "solar_cfg Write File (Section).vi"() -> ()  [unwired: 13 in, 3 out]
  n56 = call "solar_cfg Write File (Str).vi"() -> ()  [unwired: 13 in, 3 out]
  n57 = call "solar_cfg Write File (Var).vi"() -> ()  [unwired: 13 in, 3 out]
  n58 = call-poly "solar_cfg Write.vi"() -> ()  [unwired: 13 in, 3 out]
  n59 = call "solar_cfg_demo Read.vit"() -> ()  [unwired: 12 in]
  n60 = call "solar_cfg_demo Simple.vit"() -> ()  [unwired: 12 in]
  n61 = call "solar_cfg_demo Write.vit"() -> ()  [unwired: 12 in]
  n62 = call "solar_excel Cell Escape.vi"() -> ()  [unwired: 11 in, 1 out]
  n63 = call "solar_excel Cell Next.vi"() -> ()  [unwired: 8 in, 4 out]
  n64 = call "solar_excel Cell Range.vi"() -> ()  [unwired: 9 in, 3 out]
  n65 = call "solar_excel Cell String to Range.vi"() -> ()  [unwired: 11 in, 1 out]
  n66 = call "solar_excel Cell Truncate.vi"() -> ()  [unwired: 11 in, 1 out]
  n67 = call "solar_excel Cell Values (Column).vi"() -> ()  [unwired: 10 in, 2 out]
  n68 = call "solar_excel Cell Values (Row).vi"() -> ()  [unwired: 10 in, 2 out]
  n69 = call "solar_excel Cell Values.vi"() -> ()  [unwired: 9 in, 3 out]
  n70 = call "solar_excel Close.vi"() -> ()  [unwired: 11 in, 1 out]
  n71 = call "solar_excel Create.vi"() -> ()  [unwired: 10 in, 2 out]
  n72 = call "solar_excel Export.vi"() -> ()  [unwired: 10 in, 2 out]
  n73 = call "solar_excel File Read (All).vi"() -> ()  [unwired: 8 in, 4 out]
  n74 = call "solar_excel File Read (Sheet).vi"() -> ()  [unwired: 9 in, 3 out]
  n75 = call "solar_excel File Write (All).vi"() -> ()  [unwired: 10 in, 2 out]
  n76 = call "solar_excel File Write (Append Row).vi"() -> ()  [unwired: 10 in, 2 out]
  n77 = call "solar_excel File Write (Sheet).vi"() -> ()  [unwired: 10 in, 2 out]
  n78 = call "solar_excel Import.vi"() -> ()  [unwired: 10 in, 2 out]
  n79 = call "solar_excel Open.vi"() -> ()  [unwired: 10 in, 2 out]
  n80 = call "solar_excel Template.vit"() -> ()  [unwired: 11 in, 1 out]
  n81 = call "solar_excel Workbook Close.vi"() -> ()  [unwired: 10 in, 2 out]
  n82 = call "solar_excel Workbook Create.vi"() -> ()  [unwired: 10 in, 2 out]
  n83 = call "solar_excel Workbook Get Sheets.vi"() -> ()  [unwired: 8 in, 4 out]
  n84 = call "solar_excel Workbook Open.vi"() -> ()  [unwired: 10 in, 2 out]
  n85 = call "solar_excel Worksheet Build (tsv).vi"() -> ()  [unwired: 11 in, 1 out]
  n86 = call "solar_excel Worksheet Close.vi"() -> ()  [unwired: 10 in, 2 out]
  n87 = call "solar_excel Worksheet Create.vi"() -> ()  [unwired: 10 in, 2 out]
  n88 = call "solar_excel Worksheet Format (Range).vi"() -> ()  [unwired: 10 in, 2 out]
  n89 = call "solar_excel Worksheet Open.vi"() -> ()  [unwired: 8 in, 4 out]
  n90 = call "solar_excel Worksheet Parse (tsv).vi"() -> ()  [unwired: 10 in, 2 out]
  n91 = call "solar_excel Worksheet Range.vi"() -> ()  [unwired: 8 in, 4 out]
  n92 = call "solar_excel Worksheet Read (Range).vi"() -> ()  [unwired: 9 in, 3 out]
  n93 = call "solar_excel Worksheet Read (Sheet).vi"() -> ()  [unwired: 9 in, 3 out]
  n94 = call "solar_excel Worksheet Rename.vi"() -> ()  [unwired: 10 in, 2 out]
  n95 = call "solar_excel Worksheet Write (Range).vi"() -> ()  [unwired: 10 in, 2 out]
  n96 = call "solar_log Banner Dialog.vi"() -> ()  [unwired: 12 in]
  n97 = call "solar_log Banner.vi"() -> ()  [unwired: 11 in, 1 out]
  n98 = call "solar_log Create.vi"() -> ()  [unwired: 11 in, 1 out]
  n99 = call "solar_log Destroy.vi"() -> ()  [unwired: 11 in, 1 out]
  n100 = call "solar_log EnQ (Message).vi"() -> ()  [unwired: 11 in, 1 out]
  n101 = call "solar_log EnQ.vi"() -> ()  [unwired: 9 in, 3 out]
  n102 = call "solar_log Filter.vi"() -> ()  [unwired: 11 in, 1 out]
  n103 = call "solar_log Menu.vi"() -> ()  [unwired: 11 in, 1 out]
  n104 = call "solar_log New File.vi"() -> ()  [unwired: 9 in, 3 out]
  n105 = call "solar_log Variant to String.vi"() -> ()  [unwired: 9 in, 3 out]
  n106 = call "solar_log_demo.vit"() -> ()  [unwired: 12 in]
  n107 = call "solar_misc Array Duplicates.vi"() -> ()  [unwired: 10 in, 2 out]
  n108 = call "solar_misc CPU Memory.vi"() -> ()  [unwired: 7 in, 5 out]
  n109 = call "solar_misc CPU Usage.vi"() -> ()  [unwired: 9 in, 3 out]
  n110 = call "solar_misc CPU.vi"() -> ()  [unwired: 10 in, 2 out]
  n111 = call "solar_misc Create Project Tree.vi"() -> ()  [unwired: 8 in, 4 out]
  n112 = call "solar_misc Create VI Tree.vi"() -> ()  [unwired: 11 in, 1 out]
  n113 = call "solar_misc Delta Time.vi"() -> ()  [unwired: 7 in, 3 out]
  n114 = call "solar_misc Edit Help Link.vi"() -> ()  [unwired: 12 in]
  n115 = call "solar_misc Elapsed Time.vi"() -> ()  [unwired: 7 in, 3 out]
  n116 = call "solar_misc Email Config.vi"() -> ()  [unwired: 9 in, 3 out]
  n117 = call "solar_misc Email Dialog.vi"() -> ()  [unwired: 9 in, 3 out]
  n118 = call "solar_misc Email Send.vi"() -> ()  [unwired: 13 in, 3 out]
  n119 = call "solar_misc Export VIConPane Images.vi"() -> ()  [unwired: 12 in]
  n120 = call "solar_misc Generate Error.vi"() -> ()  [unwired: 12 in]
  n121 = call "solar_misc Get Bytes.vi"() -> ()  [unwired: 9 in, 3 out]
  n122 = call "solar_misc Image Overlay.vi"() -> ()  [unwired: 10 in, 2 out]
  n123 = call "solar_misc List StaticVIs.vi"() -> ()  [unwired: 9 in, 3 out]
  n124 = call "solar_misc LVClass Descendants.vi"() -> ()  [unwired: 10 in, 2 out]
  n125 = call "solar_misc LVClass Hierarchy.vi"() -> ()  [unwired: 9 in, 3 out]
  n126 = call "solar_misc LVClass List.vi"() -> ()  [unwired: 1 out]
  n127 = call "solar_misc Netstat Port Status.vi"() -> ()  [unwired: 9 in, 3 out]
  n128 = call "solar_misc Netstat Query.vi"() -> ()  [unwired: 10 in, 2 out]
  n129 = call "solar_misc Netstat.vi"() -> ()  [unwired: 12 in]
  n130 = call "solar_misc Parse CSV.vi"() -> ()  [unwired: 9 in, 1 out]
  n131 = call "solar_misc Parse TSV.vi"() -> ()  [unwired: 9 in, 1 out]
  n132 = call "solar_misc Parse WSV.vi"() -> ()  [unwired: 9 in, 1 out]
  n133 = call "solar_misc Rendezvous Create.vi"() -> ()  [unwired: 9 in, 3 out]
  n134 = call "solar_misc Rendezvous Destroy.vi"() -> ()  [unwired: 11 in, 1 out]
  n135 = call "solar_misc Rendezvous Wait.vi"() -> ()  [unwired: 9 in, 3 out]
  n136 = call "solar_misc Unix Time.vi"() -> ()  [unwired: 10 in, 2 out]
  n137 = call "solar_misc Unpack LLB.vi"() -> ()  [unwired: 12 in]
  n138 = call "solar_misc xml Attribute.vi"() -> ()  [unwired: 10 in, 2 out]
  n139 = call "solar_misc xml Escape.vi"() -> ()  [unwired: 9 in, 1 out]
  n140 = call "solar_misc xml Parse.vi"() -> ()  [unwired: 7 in, 5 out]
  n141 = call "solar_msg Q DeQ.vi"() -> ()  [unwired: 7 in, 5 out]
  n142 = call "solar_msg Q EnQ (Name).vi"() -> ()  [unwired: 8 in, 4 out]
  n143 = call "solar_msg Q EnQ.vi"() -> ()  [unwired: 9 in, 3 out]
  n144 = call "solar_msg Q Filter.vi"() -> ()  [unwired: 10 in, 2 out]
  n145 = call "solar_msg Q HS.vi"() -> ()  [unwired: 11 in, 1 out]
  n146 = call "solar_msg Q Name.vi"() -> ()  [unwired: 8 in, 2 out]
  n147 = call "solar_msg Q Obtain.vi"() -> ()  [unwired: 9 in, 3 out]
  n148 = call "solar_msg Q Release.vi"() -> ()  [unwired: 9 in, 3 out]
  n149 = call "solar_msg Q Status.vi"() -> ()  [unwired: 5 in, 7 out]
  n150 = call "solar_msg Q Wait.vi"() -> ()  [unwired: 9 in, 3 out]
  n151 = call "solar_msg Qs Shutdown.vi"() -> ()  [unwired: 10 in, 2 out]
  n152 = call "solar_msg UE Create.vi"() -> ()  [unwired: 10 in, 2 out]
  n153 = call "solar_msg UE Destroy.vi"() -> ()  [unwired: 11 in, 1 out]
  n154 = call "solar_msg UE Generate.vi"() -> ()  [unwired: 10 in, 2 out]
  n155 = call "solar_msg_cmd.vit"() -> ()  [unwired: 9 in, 3 out]
  n156 = call "solar_msg_demo Q UI.vit"() -> ()  [unwired: 12 in]
  n157 = call "solar_msg_demo Q.vit"() -> ()  [unwired: 12 in]
  n158 = call "solar_msg_demo UE.vit"() -> ()  [unwired: 12 in]
  n159 = call "solar_msg_demo.vit"() -> ()  [unwired: 12 in]
  n160 = call "solar_qtimer Create.vi"() -> ()  [unwired: 10 in, 2 out]
  n161 = call "solar_qtimer Daemon.vi"() -> ()  [unwired: 11 in, 1 out]
  n162 = call "solar_qtimer Destroy.vi"() -> ()  [unwired: 11 in, 1 out]
  n163 = call "solar_qtimer Destroy2.vi"() -> ()  [unwired: 11 in, 1 out]
  n164 = call "solar_qtimer EnQ.vi"() -> ()  [unwired: 9 in, 3 out]
  n165 = call "solar_qtimer Find.vi"() -> ()  [unwired: 10 in, 2 out]
  n166 = call "solar_qtimer Get Qtimer Names for Target.vi"() -> ()  [unwired: 11 in, 1 out]
  n167 = call "solar_qtimer Get QTimers.vi"() -> ()  [unwired: 9 in, 3 out]
  n168 = call "solar_qtimer Get.vi"() -> ()  [unwired: 9 in, 3 out]
  n169 = call "solar_qtimer Launch.vi"() -> ()  [unwired: 10 in, 2 out]
  n170 = call "solar_qtimer Obtain.vi"() -> ()  [unwired: 10 in, 2 out]
  n171 = call "solar_qtimer Process.vi"() -> ()  [unwired: 12 in]
  n172 = call "solar_qtimer Refnum QTimer to SEQ.vi"() -> ()  [unwired: 1 in, 1 out]
  n173 = call "solar_qtimer Refnum SEQ to QTimer.vi"() -> ()  [unwired: 1 in, 1 out]
  n174 = call "solar_qtimer Release.vi"() -> ()  [unwired: 10 in, 2 out]
  n175 = call "solar_qtimer Set (Delay).vi"() -> ()  [unwired: 11 in, 1 out]
  n176 = call "solar_qtimer Set (EnQType).vi"() -> ()  [unwired: 11 in, 1 out]
  n177 = call "solar_qtimer Set (Message).vi"() -> ()  [unwired: 11 in, 1 out]
  n178 = call "solar_qtimer Set (Start).vi"() -> ()  [unwired: 11 in, 1 out]
  n179 = call "solar_qtimer Set Delay.vi"() -> ()  [unwired: 10 in, 2 out]
  n180 = call "solar_qtimer Set EnQType.vi"() -> ()  [unwired: 10 in, 2 out]
  n181 = call "solar_qtimer Set Messages.vi"() -> ()  [unwired: 10 in, 2 out]
  n182 = call "solar_qtimer Set Start Target.vi"() -> ()  [unwired: 8 in, 4 out]
  n183 = call "solar_qtimer Set Start.vi"() -> ()  [unwired: 10 in, 2 out]
  n184 = call "solar_qtimer Set Stop All.vi"() -> ()  [unwired: 8 in, 4 out]
  n185 = call "solar_qtimer Set Stop Target.vi"() -> ()  [unwired: 8 in, 4 out]
  n186 = call "solar_qtimer Set.vi"() -> ()  [unwired: 10 in, 2 out]
  n187 = call "solar_qtimer_demo 2.vit"() -> ()  [unwired: 12 in]
  n188 = call "solar_qtimer_demo.vit"() -> ()  [unwired: 12 in]
  n189 = call "solar Ctrls Load.vi"() -> ()  [unwired: 10 in, 2 out]
  n190 = call "solar Ctrls Save.vi"() -> ()  [unwired: 9 in, 3 out]
  n191 = call "solar Delete COSMOS Files.vi"() -> ()  [unwired: 11 in, 1 out]
  n192 = call "solar Delete Target COSMOS Files.vi"() -> ()  [unwired: 10 in, 2 out]
  n193 = call "solar Destroy (Targets).vi"() -> ()  [unwired: 11 in, 1 out]
  n194 = call "solar Exit (Children).vi"() -> ()  [unwired: 10 in, 2 out]
  n195 = call "solar Find (Target).vi"() -> ()  [unwired: 10 in, 2 out]
  n196 = call "solar Hide Packets.vi"() -> ()  [unwired: 10 in, 2 out]
  n197 = call "solar Menu (Handle).vi"() -> ()  [unwired: 11 in, 1 out]
  n198 = call "solar Menu (Initialize).vi"() -> ()  [unwired: 11 in, 1 out]
  n199 = call "solar Menu TargetsLB.vi"() -> ()  [unwired: 11 in, 1 out]
  n200 = call "solar Msg EnQ (Main).vi"() -> ()  [unwired: 9 in, 3 out]
  n201 = call "solar Msg EnQ (This).vi"() -> ()  [unwired: 9 in, 3 out]
  n202 = call "solar Msg Other (Broadcast).vi"() -> ()  [unwired: 10 in, 2 out]
  n203 = call "solar Msg Other (TLM-Broadcast).vi"() -> ()  [unwired: 10 in, 2 out]
  n204 = call "solar Msg UE Generate.vi"() -> ()  [unwired: 10 in, 2 out]
  n205 = call "solar Msg UE Main Generate.vi"() -> ()  [unwired: 10 in, 2 out]
  n206 = call "solar Msg Voyager (HS).vi"() -> ()  [unwired: 10 in, 2 out]
  n207 = call "solar Msg Voyager (Packet).vi"() -> ()  [unwired: 10 in, 2 out]
  n208 = call "solar Msg Voyager (Relay).vi"() -> ()  [unwired: 10 in, 2 out]
  n209 = call "solar Msg Voyager (TLM).vi"() -> ()  [unwired: 10 in, 2 out]
  n210 = call-poly "solar Msg.vi"() -> ()  [unwired: 9 in, 3 out]
  n211 = call "solar QTimers Launch.vi"() -> ()  [unwired: 10 in, 2 out]
  n212 = call "solar Refnum Type Cast (From).vi"() -> ()  [unwired: 1 in, 1 out]
  n213 = call "solar Refnum Type Cast (Preview).vi"() -> ()  [unwired: 9 in, 1 out]
  n214 = call "solar Refnum Type Cast (To).vi"() -> ()  [unwired: 1 in, 1 out]
  n215 = call "solar Target by Name.vi"() -> ()  [unwired: 10 in, 2 out]
  n216 = call "solar Voyager Launch Single Target.vi"() -> ()  [unwired: 10 in, 2 out]
  n217 = call "solar Voyager Launch.vi"() -> ()  [unwired: 10 in, 2 out]
  n218 = call "solar_write LogPause.vi"() -> ()  [unwired: 10 in, 2 out]
  n219 = call "solar_write LogRestart.vi"() -> ()  [unwired: 10 in, 2 out]
  n220 = call "solar_write LogWrite.vi"() -> ()  [unwired: 10 in, 2 out]
  n221 = call "solar_read MainIsMain.vi"() -> ()  [unwired: 9 in, 3 out]
  n222 = call "solar_read MainName.vi"() -> ()  [unwired: 9 in, 3 out]
  n223 = call "solar_read MainQ.vi"() -> ()  [unwired: 9 in, 3 out]
  n224 = call "solar_read MainUE.vi"() -> ()  [unwired: 9 in, 3 out]
  n225 = call "solar_write QTimerAdd.vi"() -> ()  [unwired: 10 in, 2 out]
  n226 = call "solar_read QTimerNames.vi"() -> ()  [unwired: 9 in, 3 out]
  n227 = call "solar_read QTimerQTimers.vi"() -> ()  [unwired: 9 in, 3 out]
  n228 = call "solar_read QTimerRefnum.vi"() -> ()  [unwired: 9 in, 3 out]
  n229 = call "solar_write QTimerStart.vi"() -> ()  [unwired: 10 in, 2 out]
  n230 = call "solar_write QTimerStartTarget.vi"() -> ()  [unwired: 10 in, 2 out]
  n231 = call "solar_write QTimerStop.vi"() -> ()  [unwired: 10 in, 2 out]
  n232 = call "solar_write QTimerStopAll.vi"() -> ()  [unwired: 9 in, 3 out]
  n233 = call "solar_write QTimerStopTarget.vi"() -> ()  [unwired: 10 in, 2 out]
  n234 = call "solar_read SOLARAppInfo.vi"() -> ()  [unwired: 9 in, 3 out]
  n235 = call "solar_read SOLARUE.vi"() -> ()  [unwired: 9 in, 3 out]
  n236 = call "solar_write SOLARUE_MSG.vi"() -> ()  [unwired: 10 in, 2 out]
  n237 = call "solar_write SOLARUIActive.vi"() -> ()  [unwired: 10 in, 2 out]
  n238 = call "solar_write SOLARUIHide.vi"() -> ()  [unwired: 10 in, 2 out]
  n239 = call "solar_write SOLARUIPanes.vi"() -> ()  [unwired: 10 in, 2 out]
  n240 = call "solar_write SOLARUIRefresh.vi"() -> ()  [unwired: 10 in, 2 out]
  n241 = call "solar_write SOLARUIUnhide.vi"() -> ()  [unwired: 10 in, 2 out]
  n242 = call "solar_write SOLARUIUnpin.vi"() -> ()  [unwired: 10 in, 2 out]
  n243 = call "solar_write SubscribeThisQ.vi"() -> ()  [unwired: 10 in, 2 out]
  n244 = call "solar_write SubscribeThisUE.vi"() -> ()  [unwired: 10 in, 2 out]
  n245 = call "solar_read SOLARTargets.vi"() -> ()  [unwired: 9 in, 3 out]
  n246 = call "solar_read SOLARTargetsNames.vi"() -> ()  [unwired: 9 in, 3 out]
  n247 = call "solar_read ThisBroadcastQs.vi"() -> ()  [unwired: 9 in, 3 out]
  n248 = call "solar_read ThisBroadcastUEs.vi"() -> ()  [unwired: 9 in, 3 out]
  n249 = call "solar_read ThisCtrls.vi"() -> ()  [unwired: 9 in, 3 out]
  n250 = call "solar_write ThisCtrls.vi"() -> ()  [unwired: 10 in, 2 out]
  n251 = call "solar_read ThisData.vi"() -> ()  [unwired: 9 in, 3 out]
  n252 = call "solar_write ThisData.vi"() -> ()  [unwired: 10 in, 2 out]
  n253 = call "solar_read ThisHS.vi"() -> ()  [unwired: 9 in, 3 out]
  n254 = call "solar_write ThisHS.vi"() -> ()  [unwired: 10 in, 2 out]
  n255 = call "solar_read ThisIni.vi"() -> ()  [unwired: 9 in, 3 out]
  n256 = call "solar_read ThisLogIgnore.vi"() -> ()  [unwired: 9 in, 3 out]
  n257 = call "solar_write ThisLogIgnore.vi"() -> ()  [unwired: 10 in, 2 out]
  n258 = call "solar_read ThisName.vi"() -> ()  [unwired: 9 in, 3 out]
  n259 = call "solar_read ThisQ.vi"() -> ()  [unwired: 9 in, 3 out]
  n260 = call "solar_read ThisUE.vi"() -> ()  [unwired: 9 in, 3 out]
  n261 = call "solar_read ThisVI.vi"() -> ()  [unwired: 9 in, 3 out]
  n262 = call "solar_write UnsubscribeThisQ.vi"() -> ()  [unwired: 10 in, 2 out]
  n263 = call "solar_write UnsubscribeThisUE.vi"() -> ()  [unwired: 10 in, 2 out]
  n264 = call "solar_write VoyagerExport.vi"() -> ()  [unwired: 10 in, 2 out]
  n265 = call "solar_read VoyagerPackets.vi"() -> ()  [unwired: 9 in, 3 out]
  n266 = call "solar_write VoyagerPackets.vi"() -> ()  [unwired: 10 in, 2 out]
  n267 = call "solar_write VoyagerPacketsOverride.vi"() -> ()  [unwired: 10 in, 2 out]
  n268 = call "solar_write VoyagerRefnum.vi"() -> ()  [unwired: 10 in, 2 out]
  n269 = call "solar_read VoyagerRefnum.vi"() -> ()  [unwired: 9 in, 3 out]
  n270 = call "solar_probe.vi"() -> ()  [unwired: 10 in, 2 out]
  n271 = call "solar Build INI Path.vi"() -> ()  [unwired: 10 in, 2 out]
  n272 = call-dynamic "solar Command.vi"() -> ()  [unwired: 7 in, 5 out]
  n273 = call "solar Create (Addons).vi"() -> ()  [unwired: 10 in, 2 out]
  n274 = call "solar Create (Application).vi"() -> ()  [unwired: 10 in, 2 out]
  n275 = call "solar Create (LVClass).vi"() -> ()  [unwired: 9 in, 3 out]
  n276 = call "solar Create (LVClass.ini).vi"() -> ()  [unwired: 9 in, 3 out]
  n277 = call "solar Create (SOLAR).vi"() -> ()  [unwired: 10 in, 2 out]
  n278 = call "solar Create (Target).vi"() -> ()  [unwired: 10 in, 2 out]
  n279 = call "solar Create.vi"() -> ()  [unwired: 8 in, 4 out]
  n280 = call "solar DeQ.vi"() -> ()  [unwired: 7 in, 5 out]
  n281 = call "solar Destroy.vi"() -> ()  [unwired: 11 in, 1 out]
  n282 = call-dynamic "solar Error Handle.vi"() -> ()  [unwired: 9 in, 3 out]
  n283 = call-dynamic "solar Exit.vi"() -> ()  [unwired: 9 in, 3 out]
  n284 = call "solar Handshake.vi"() -> ()  [unwired: 10 in, 2 out]
  n285 = call-dynamic "solar Initialize.vi"() -> ()  [unwired: 10 in, 2 out]
  n286 = call-dynamic "solar Interlocks.vi"() -> ()  [unwired: 8 in, 4 out]
  n287 = call "solar Log.vi"() -> ()  [unwired: 10 in, 2 out]
  n288 = call "solar Menu.vi"() -> ()  [unwired: 10 in, 2 out]
  n289 = call-dynamic "solar Pack.vi"() -> ()  [unwired: 8 in, 4 out]
  n290 = call-dynamic "solar Private Data.vi"() -> ()  [unwired: 10 in, 2 out]
  n291 = call-dynamic "solar Register.vi"() -> ()  [unwired: 10 in, 2 out]
  n292 = call-dynamic "solar Rendezvous.vi"() -> ()  [unwired: 8 in, 4 out]
  n293 = call-dynamic "solar Setup.vi"() -> ()  [unwired: 10 in, 2 out]
  n294 = call-dynamic "solar Teardown.vi"() -> ()  [unwired: 10 in, 2 out]
  n295 = call-dynamic "solar Unpack.vi"() -> ()  [unwired: 8 in, 4 out]
  n296 = call "solar_gbl Create Refnums.vi"() -> ()  [unwired: 8 in, 4 out]
  n297 = call "solar_gbl Launch Splash.vi"() -> ()  [unwired: 9 in, 3 out]
  n298 = call "solar_gbl Launch Targets.vi"() -> ()  [unwired: 9 in, 3 out]
  n299 = call "solar_gbl Read Config (Override).vi"() -> ()  [unwired: 8 in, 4 out]
  n300 = call "solar_gbl Read Config.vi"() -> ()  [unwired: 8 in, 4 out]
  n301 = call "solar_ui Active.vi"() -> ()  [unwired: 10 in, 2 out]
  n302 = call "solar_ui Listbox Initialize.vi"() -> ()  [unwired: 6 in, 6 out]
  n303 = call "solar_ui Listbox.vi"() -> ()  [unwired: 9 in, 3 out]
  n304 = call "solar_ui Resize.vi"() -> ()  [unwired: 11 in, 1 out]
  n305 = call "solar_ui Unpin.vi"() -> ()  [unwired: 9 in, 3 out]
  n306 = call "solar_ui.vi"() -> ()  [unwired: 12 in]
  n307 = call "solar_tcp Bits Get.vi"() -> ()  [unwired: 9 in, 3 out]
  n308 = call "solar_tcp Bits Set.vi"() -> ()  [unwired: 11 in, 1 out]
  n309 = call "solar_tcp Close.vi"() -> ()  [unwired: 10 in, 2 out]
  n310 = call "solar_tcp Config.vi"() -> ()  [unwired: 9 in, 3 out]
  n311 = call "solar_tcp Core Client.vi"() -> ()  [unwired: 8 in, 4 out]
  n312 = call "solar_tcp Core Server.vi"() -> ()  [unwired: 8 in, 4 out]
  n313 = call "solar_tcp Core.vi"() -> ()  [unwired: 8 in, 4 out]
  n314 = call "solar_tcp Debug Get.vi"() -> ()  [unwired: 9 in, 3 out]
  n315 = call "solar_tcp Debug Set.vi"() -> ()  [unwired: 10 in, 2 out]
  n316 = call "solar_tcp Generate Error.vi"() -> ()  [unwired: 11 in, 1 out]
  n317 = call "solar_tcp Identify.vi"() -> ()  [unwired: 8 in, 4 out]
  n318 = call "solar_tcp Open.vi"() -> ()  [unwired: 9 in, 3 out]
  n319 = call "solar_tcp Read.vi"() -> ()  [unwired: 8 in, 4 out]
  n320 = call "solar_tcp Write.vi"() -> ()  [unwired: 8 in, 4 out]
  n321 = call "solar_tcp_demo Example.vit"() -> ()  [unwired: 12 in]
  n322 = call "solar_tcp_demo.vit"() -> ()  [unwired: 12 in]
  n323 = call "solar_type Get Bits.vi"() -> ()  [unwired: 9 in, 3 out]
  n324 = call "solar_type Get Items (Ctrl).vi"() -> ()  [unwired: 7 in, 5 out]
  n325 = call "solar_type Get Items (Variants).vi"() -> ()  [unwired: 8 in, 4 out]
  n326 = call "solar_type Get Type.vi"() -> ()  [unwired: 5 in, 3 out]
  n327 = call "solar_type Get Value (ASCII).vi"() -> ()  [unwired: 9 in, 3 out]
  n328 = call "solar_type Get Value (Binary).vi"() -> ()  [unwired: 7 in, 5 out]
  n329 = call "solar_type Message to Script.vi"() -> ()  [unwired: 10 in, 2 out]
  n330 = call "solar_type Script to Message.vi"() -> ()  [unwired: 6 in, 6 out]
  n331 = call "solar_type Script to Messages.vi"() -> ()  [unwired: 8 in, 4 out]
  n332 = call "solar_type Script Type to Variant.vi"() -> ()  [unwired: 8 in, 4 out]
  n333 = call "solar_type Set Bits.vi"() -> ()  [unwired: 11 in, 1 out]
  n334 = call "solar_type Set Items (Types).vi"() -> ()  [unwired: 10 in, 2 out]
  n335 = call "solar_type Set Items (Variants).vi"() -> ()  [unwired: 10 in, 2 out]
  n336 = call "solar_type Set Type.vi"() -> ()  [unwired: 8 in, 2 out]
  n337 = call "solar_type Set Value (ASCII).vi"() -> ()  [unwired: 9 in, 3 out]
  n338 = call "solar_type Set Variant.vi"() -> ()  [unwired: 9 in, 3 out]
  n339 = call "solar_type Variant Array to Cluster.vi"() -> ()  [unwired: 11 in, 1 out]
  n340 = call "solar_type Variant Set Enum Names.vi"() -> ()  [unwired: 10 in, 2 out]
  n341 = call "solar_type Variant to Arguments.vi"() -> ()  [unwired: 9 in, 1 out]
  n342 = call "solar_visa Query (Simulate).vi"() -> ()  [unwired: 9 in, 3 out]
  n343 = call "solar_visa VISA Close.vi"() -> ()  [unwired: 10 in, 2 out]
  n344 = call "solar_visa VISA Open.vi"() -> ()  [unwired: 10 in, 2 out]
  n345 = call "solar_visa VISA Query (Error).vi"() -> ()  [unwired: 10 in, 2 out]
  n346 = call "solar_visa VISA Query.vi"() -> ()  [unwired: 8 in, 4 out]
  n347 = call "solar_visa VISA Timeout.vi"() -> ()  [unwired: 9 in, 3 out]
  n348 = call "solar_visa_demo.vit"() -> ()  [unwired: 12 in]
  n349 = call "solar_voy Packet Unpack.vi"() -> ()  [unwired: 8 in, 4 out]
  n350 = call "solar_voy_def Display Tree.vi"() -> ()  [unwired: 11 in, 1 out]
  n351 = call "solar_voy_def Export (cmd_tlm).vi"() -> ()  [unwired: 10 in, 2 out]
  n352 = call "solar_voy_def Export (cmd_tlm_server).vi"() -> ()  [unwired: 9 in, 3 out]
  n353 = call "solar_voy_def Export (cosmos).vi"() -> ()  [unwired: 10 in, 2 out]
  n354 = call "solar_voy_def Export (Interface_LINC).vi"() -> ()  [unwired: 11 in, 1 out]
  n355 = call "solar_voy_def Export (Item).vi"() -> ()  [unwired: 9 in, 3 out]
  n356 = call "solar_voy_def Export (Mods).vi"() -> ()  [unwired: 11 in, 1 out]
  n357 = call "solar_voy_def Export (Mods_Convert).vi"() -> ()  [unwired: 11 in, 1 out]
  n358 = call "solar_voy_def Export (Mods_Limits).vi"() -> ()  [unwired: 11 in, 1 out]
  n359 = call "solar_voy_def Export (Mods_State).vi"() -> ()  [unwired: 11 in, 1 out]
  n360 = call "solar_voy_def Export (Packet).vi"() -> ()  [unwired: 8 in, 4 out]
  n361 = call "solar_voy_def Export (Packets).vi"() -> ()  [unwired: 10 in, 2 out]
  n362 = call "solar_voy_def Export (Targets).vi"() -> ()  [unwired: 8 in, 4 out]
  n363 = call "solar_voy_def Export Type.vi"() -> ()  [unwired: 14 in, 2 out]
  n364 = call "solar_voy_def Export Value.vi"() -> ()  [unwired: 15 in, 1 out]
  n365 = call-poly "solar_voy_def Export.vi"() -> ()  [unwired: 10 in, 2 out]
  n366 = call "solar_voy_def Find Item (Name).vi"() -> ()  [unwired: 11 in, 1 out]
  n367 = call "solar_voy_def Find Packet (ID).vi"() -> ()  [unwired: 11 in, 1 out]
  n368 = call "solar_voy_def Find Packet (Name).vi"() -> ()  [unwired: 11 in, 1 out]
  n369 = call "solar_voy_def GUID.vi"() -> ()  [unwired: 8 in, 4 out]
  n370 = call "solar_voy_def HS_DATA.vi"() -> ()  [unwired: 11 in, 1 out]
  n371 = call "solar_voy_def Import (cmd_tlm).vi"() -> ()  [unwired: 10 in, 2 out]
  n372 = call "solar_voy_def Import (cmd_tlm_server).vi"() -> ()  [unwired: 10 in, 2 out]
  n373 = call "solar_voy_def Import (Empty).vi"() -> ()  [unwired: 10 in, 2 out]
  n374 = call "solar_voy_def Import (Header).vi"() -> ()  [unwired: 10 in, 2 out]
  n375 = call "solar_voy_def Import (Item_Def).vi"() -> ()  [unwired: 9 in, 3 out]
  n376 = call "solar_voy_def Import (Refnum).vi"() -> ()  [unwired: 10 in, 2 out]
  n377 = call "solar_voy_def Import (Required).vi"() -> ()  [unwired: 10 in, 2 out]
  n378 = call "solar_voy_def Import (Simple).vi"() -> ()  [unwired: 10 in, 2 out]
  n379 = call "solar_voy_def Import (Variant).vi"() -> ()  [unwired: 10 in, 2 out]
  n380 = call "solar_voy_def Import (Variants).vi"() -> ()  [unwired: 10 in, 2 out]
  n381 = call-poly "solar_voy_def Import.vi"() -> ()  [unwired: 10 in, 2 out]
  n382 = call "solar_voy_def Items Bit Offsets.vi"() -> ()  [unwired: 10 in, 2 out]
  n383 = call "solar_voy_def Items Bit Size.vi"() -> ()  [unwired: 10 in, 2 out]
  n384 = call "solar_voy_def LVType to Type.vi"() -> ()  [unwired: 9 in, 3 out]
  n385 = call "solar_voy_def Parse Args (Desc).vi"() -> ()  [unwired: 11 in, 1 out]
  n386 = call "solar_voy_def Parse Args (Label).vi"() -> ()  [unwired: 11 in, 1 out]
  n387 = call "solar_voy_def Parse Args.vi"() -> ()  [unwired: 11 in, 1 out]
  n388 = call "solar_voy_def Quotes Add Desc.vi"() -> ()  [unwired: 11 in, 1 out]
  n389 = call "solar_voy_def Quotes Add LVType.vi"() -> ()  [unwired: 11 in, 1 out]
  n390 = call "solar_voy_def Quotes Add.vi"() -> ()  [unwired: 11 in, 1 out]
  n391 = call "solar_voy_def Quotes Remove.vi"() -> ()  [unwired: 11 in, 1 out]
  n392 = call "solar_voy_def Rename Channels.vi"() -> ()  [unwired: 10 in, 2 out]
  n393 = call "solar_voy_def Rename Packet.vi"() -> ()  [unwired: 10 in, 2 out]
  n394 = call "solar_voy_def Resolve ASCII (Default).vi"() -> ()  [unwired: 11 in, 1 out]
  n395 = call "solar_voy_def Resolve ASCII (Hex).vi"() -> ()  [unwired: 11 in, 1 out]
  n396 = call "solar_voy_def Resolve IDs.vi"() -> ()  [unwired: 11 in, 1 out]
  n397 = call "solar_voy_def Resolve Path.vi"() -> ()  [unwired: 10 in, 2 out]
  n398 = call "solar_voy_def Strip Description.vi"() -> ()  [unwired: 10 in, 2 out]
  n399 = call "solar_voy_def Variant Array to Cluster.vi"() -> ()  [unwired: 11 in, 1 out]
  n400 = call "solar_voy_def Variant Create.vi"() -> ()  [unwired: 10 in, 2 out]
  n401 = call "solar_voy_def Variant Get TCP.vi"() -> ()  [unwired: 9 in, 3 out]
  n402 = call "solar_voy Check Voy Header IDs.vi"() -> ()  [unwired: 10 in, 2 out]
  n403 = call "solar_voy Create.vi"() -> ()  [unwired: 9 in, 3 out]
  n404 = call "solar_voy Destroy.vi"() -> ()  [unwired: 11 in, 1 out]
  n405 = call "solar_voy EnQ (Error).vi"() -> ()  [unwired: 10 in, 2 out]
  n406 = call "solar_voy EnQ (ID).vi"() -> ()  [unwired: 10 in, 2 out]
  n407 = call "solar_voy Export.vi"() -> ()  [unwired: 10 in, 2 out]
  n408 = call "solar_voy Get Bits (COSMOS).vi"() -> ()  [unwired: 10 in, 2 out]
  n409 = call "solar_voy Get Bits (Variant).vi"() -> ()  [unwired: 8 in, 4 out]
  n410 = call "solar_voy Get Info (SEQ).vi"() -> ()  [unwired: 9 in, 3 out]
  n411 = call "solar_voy Get Info.vi"() -> ()  [unwired: 9 in, 3 out]
  n412 = call "solar_voy HS DB.vi"() -> ()  [unwired: 11 in, 5 out]
  n413 = call "solar_voy Launch.vi"() -> ()  [unwired: 10 in, 2 out]
  n414 = call "solar_voy Obtain.vi"() -> ()  [unwired: 9 in, 3 out]
  n415 = call "solar_voy Pack (HDR).vi"() -> ()  [unwired: 9 in, 3 out]
  n416 = call "solar_voy Pack.vi"() -> ()  [unwired: 12 in, 4 out]
  n417 = call "solar_voy Packets Tree.vi"() -> ()  [unwired: 10 in, 2 out]
  n418 = call "solar_voy Read Voyager ID Offset.vi"() -> ()  [unwired: 10 in, 2 out]
  n419 = call "solar_voy Refnum SEQ to Voyager.vi"() -> ()  [unwired: 1 in, 1 out]
  n420 = call "solar_voy Refnum Voyager to SEQ.vi"() -> ()  [unwired: 1 in, 1 out]
  n421 = call "solar_voy Register (Hide).vi"() -> ()  [unwired: 10 in, 2 out]
  n422 = call "solar_voy Register (Import).vi"() -> ()  [unwired: 10 in, 2 out]
  n423 = call "solar_voy Register (Packet).vi"() -> ()  [unwired: 10 in, 2 out]
  n424 = call "solar_voy Register (Packets).vi"() -> ()  [unwired: 10 in, 2 out]
  n425 = call "solar_voy Register (Required).vi"() -> ()  [unwired: 10 in, 2 out]
  n426 = call "solar_voy Release.vi"() -> ()  [unwired: 10 in, 2 out]
  n427 = call "solar_voy Set Bits (COSMOS).vi"() -> ()  [unwired: 9 in, 3 out]
  n428 = call "solar_voy Set Bits (HDR_LENGTH).vi"() -> ()  [unwired: 10 in, 2 out]
  n429 = call "solar_voy Set VI Control.vi"() -> ()  [unwired: 11 in, 1 out]
  n430 = call "solar_voy TCP Close.vi"() -> ()  [unwired: 10 in, 2 out]
  n431 = call "solar_voy TCP Listener Create.vi"() -> ()  [unwired: 9 in, 3 out]
  n432 = call "solar_voy TCP Listener Wait.vi"() -> ()  [unwired: 9 in, 3 out]
  n433 = call "solar_voy TCP Open.vi"() -> ()  [unwired: 9 in, 3 out]
  n434 = call "solar_voy TCP Process.vi"() -> ()  [unwired: 12 in]
  n435 = call "solar_voy TCP Read.vi"() -> ()  [unwired: 8 in, 4 out]
  n436 = call "solar_voy Unpack.vi"() -> ()  [unwired: 9 in, 7 out]
  n437 = call "solar_voy Valid Refnum.vi"() -> ()  [unwired: 1 in, 1 out]
  n438 = call "solar_voy VoyagerIDOffset Lookup.vi"() -> ()  [unwired: 9 in, 3 out]
  n439 = call "solar_voy Write (Handshake).vi"() -> ()  [unwired: 10 in, 2 out]
  n440 = call "solar_voy Write (HS).vi"() -> ()  [unwired: 10 in, 2 out]
  n441 = call "solar_voy Write (Relay).vi"() -> ()  [unwired: 10 in, 2 out]
  n442 = call "solar_voy Write (TCP).vi"() -> ()  [unwired: 9 in, 3 out]
  n443 = call "solar_voy Write (Variant).vi"() -> ()  [unwired: 10 in, 2 out]
  n444 = call "solar_voy Write IDOffset.vi"() -> ()  [unwired: 10 in, 2 out]
  n445 = call "solar_voy_demo Test Packets.vi"() -> ()  [unwired: 12 in]
  n446 = call "solar_voyager.vit"() -> ()  [unwired: 12 in]
  n447 = call "solar_target.vi"() -> ()  [unwired: 12 in]
  n448 = call "solar_target2.vi"() -> ()  [unwired: 12 in]
